vi "UHR-Fleezers Control (fpga) - Leonardo 04-2018 V5.3.vi"() -> ()   [LabVIEW 2013]
doc: "UHR-Fleezers Instrument Control Code (fpga)"
uses:
  <vilib>/Platform/TimedLoop/XDataNode/timing_clust.ctl
  <vilib>/Platform/TimedLoop/XDataNode/nitl_modes.ctl
  <vilib>/Platform/TimedLoop/XDataNode/wakeup.ctl
  <vilib>/rvi/eio/common/nirviEmuTemplateMethod_errors.vi
  <vilib>/rvi/Emulation/niFpgaSctlEmulationGetInTimedLoop.vi
  <vilib>/rvi/Emulation/niFpgaEmulationReportErrorSimple.vi
  <vilib>/rvi/Emulation/niFpgaGetClockAttributes.vi
  <vilib>/rvi/Emulation/niFpgaCriticalErrorInLSC.vi
  <vilib>/rvi/FIFO/Fifo_Resource/nirvififoEmulationReadFpgaImpl.vi
  <vilib>/rvi/DataTransferAndStorage/Container/Common/niFpgaContainerGetUniqueNameForEmu.vi
  <vilib>/rvi/DataTransferAndStorage/Container/Common/niFpgaContainerExecOnDevCompGetState.vi
  <vilib>/rvi/interface/RandomDataEmulation/nirviRandomDataFPGAFIFO.vi
  <vilib>/rvi/interface/RandomDataEmulation/niFpgaRandomDataHandleErrors.vi
  <vilib>/rvi/eio/common/nirviEmuReportErrorAndStop.vi
  <vilib>/rvi/Emulation/niFpgaProcessEmulError.vi
  <vilib>/rvi/FIFO/Fifo_Resource/nirvififoEmulationWriteFpgaImpl.vi
  <vilib>/Platform/TimedLoop/XDataNode/XDataNode.xnode
  <vilib>/eio/EIOMethodNode/EIOMethodNode.xnode
  <vilib>/eio/EIONode/EIONode.xnode
  <vilib>/rvi/DataTransferAndStorage/Container/XNode/niFpgaContainer.xnode
  <vilib>/rvi/FIFO/Fifo_Resource/nirvififoEmulationRead.vi
  <vilib>/rvi/FIFO/Fifo_Resource/niFpgaFifoEmulationRefIn.vi
  <vilib>/rvi/interface/RandomDataEmulation/nirviRandomDataFpgaReadWriteTemplate.vi
  <vilib>/rvi/FIFO/Fifo_Resource/nirvififoEmulationWrite.vi
  <vilib>/addons/control/pid/fpga.llb/XNode/niFpgaPID.xnode
  <vilib>/Platform/TimedLoop/XDataNode/XDNodeRunTimeDep.lvlib
  <vilib>/rvi/Memory/Memory_Emulation/niFpgaMemoryEmulationRefIn.vi
panel:
  in  "Tab Control 2":T1(tab)
  out "BD1 amplitude 1 out":u16
  out "BD1 amplitude 2 out":u16
  in  "FB output range":cluster{"output low":i16, "output high":i16}={"output low"=0, "output high"=3000}
  in  "FB Gains":T2={"proportional gain (Kc)"=10, "integral gain (Kc*Ts/Ti)"=5, "derivative gain (Kc*Td/Ts)"=0}
  in  "RF synth green feedback max":i16=4000
  in  "RD":bool=TRUE
  in  "Swap F1 and F2":bool
  in  "Scan BD":bool
  in  "Start scan":bool
  in  "OSK Bd 1":bool
  in  "Reset Bd 1":bool
  in  "PMODE":bool=TRUE
  in  "Number Interlace Cycles":u8=2 min=1 max=3
  in  "Interlace Off Parameters":u8=1 min=1 max=3
  in  "Interlace ON/OFF":bool
  out "DIO Relative phase":i16
  in  "Phase count adjustment (DIO)":i16
  in  "+ phase (DIO)":bool
  out "DIO Late Counter":u8
  in  "DIO count 1 (ticks)":u16=400
  in  "DIO count 2 (ticks)":u16=400
  in  "DIO count 3 (ticks)":u16=400
  out "AI2 Y Sum Set 2":i16
  out "AI2 Y Sum Set 1":i16
  in  "FB Setpoint Set 1":i16 min=0 step=1
  in  "FB Reset Set 1":bool
  in  "FB On/Off Set 1":bool
  in  "FB Reset Set 2":bool
  in  "FB On/Off Set 2":bool
  in  "FB Setpoint Set 2":i16 min=0 step=1
  in  "Amp switch delay":u8=5
  in  "RF synth bd controls green":bool
  in  "Phase Trap 2":fxp<+,14,14>
  in  "Phase Trap 1":fxp<+,14,14>
  in  "Phase offset method":u8
  in  "BD 2 Amplitude 1":u16
  in  "BD 1 Amplitude 1":u16
  in  "BD 2 Frequency 1":u64
  in  "BD 1 Frequency 1":u64
  in  "BD 2 Amplitude 2":u16
  in  "BD 1 Amplitude 2":u16
  in  "BD 2 Frequency 2":u64
  in  "BD 1 Frequency 2":u64
  in  "BD 2 Amplitude 3":u16
  in  "BD 1 Amplitude 3":u16
  in  "BD 2 Frequency 3":u64
  in  "BD 1 Frequency 3":u64
  in  "BD 2 Delay (Ticks)":u8 caption="Count(Ticks)"
  in  "Next trap write delay (ticks)":u8 caption="Count(Ticks)"
  out "Random phase generated":fxp<+,14,14>
  in  "RF phase reset before cycles":bool
  in  "Trap 1 osc enable":bool
  in  "N trap osc periods":i16
  in  "Trap osc period (pts)":i16
  in  "Osc traps":bool
  in  "Initiate trap osc":bool
  in  "Ready Write":bool
  in  "Data":i64
  in  "Address 2":u32
  in  "Osc trap cont.":bool
  in  "Trap 2 osc enable":bool
  out "green FB running":bool
  in  "APD 2 AO scale factor":i16=1
  in  "BD 1 Delay (ticks)":u8
  in  "Tab Control":T3(tab)=enum."MCL trap control"
  in  "Set 3":bool
  in  "Set 2":bool=TRUE
  in  "Set 1":bool=TRUE
  in  "Trap Pos to FIFO":bool
  in  "N of AI1 Int Acq Sets":i16=2 min=1 max=3 step=1
  out "AI Late Counter":u8
  in  "ai count":u16=400
  in  "+ phase":bool
  in  "Phase count adjustment":i16
  out "Relative phase":i16
  in  "AI to FIFO":bool
  out "BD1 Frequency Out 1":u64
  out "BD1 Frequency Out 2":u64
  out "Trap Pos FIFO Timeout":u16
  out "Trap AI FIFO Timeout":u16
  in  "Trap FIFO Set Timeout":i32
  in  "Scan freq.  increment":i64
  in  "Scan steps":u64
  in  "Number of scans":u16
  in  "Cycles per step":u64
  in  "Raster setpoint":fxp<+/-,16,1>
  in  "Raster to target force":bool
  out "Actual Scan freq":u64
  in  "Cont. Scan":bool
  out "Scan I":u64
  in  "Abort scan":bool
  out "Scanning":bool
  in  "Symmetric FB/Raster":bool
  in  "FB Min frequency":u64
  in  "FB Max Frequency":u64
  in  "Dynamic Force FB (Ronen)":bool
  in  "Trap pos. FB Range":T4={"FB2 output low"=-1.0, "FB2 output high"=0.999969482421875}
  in  "Trap Pos. FB Gains":T5={"proportional gain (Kc)"=0.999969482421875, "integral gain (Kc*Ts/Ti)"=0.999969482421875, "derivative gain (Kc*Td/Ts)"=0.0}
  in  "B factor":fxp<+/-,32,16>
  in  "Negate Diff?":bool
  in  "Diff FB Measurement?":bool
  in  "FB Trig Integrate":u32=1
  out "TTrig?":bool
  in  "TTrig Negate Pos":bool=TRUE
  out "Trap Pos FB Int Signal":fxp<+/-,24,9> format="%.18g"
  out "Trap Pos FB Int-Norm Signal":fxp<+/-,16,1> format="%.16g"
  in  "FPGA TTrig Thresh":i64
  in  "FPGA Trap Trig":bool
  out "Trap Pos FB Action":i64
  in  "Trap Pos. FB Offset Factor":i64
  in  "Trap Pos. FB Mult Factor":i64=2
  in  "Trap Pos. FB Reset":bool
  in  "Trap Pos FB Monitor T1 or T2":bool
  in  "AI1 X Scale":u16
  in  "Trap Pos FB Int Count":u16=100
  in  "Trap Pos FB Negate Action":bool
  out "AI1 X Set 2":fxp<+/-,16,1>
  out "AI1 X Set 1":fxp<+/-,16,1>
  in  "Trap Pos. FB SP":fxp<+/-,16,1>
  in  "Force feedback":bool
  out "TTrig Sig":i64
  out "TTrig Fin Thresh":i64
  in  "1D or 2D Scan?":bool
  in  "Abort scan (MCL)":bool
  in  "MCL Scan Axis":bool
  in  "Cont. Scan (MCL)":bool
  out "Scan I (MCL)":u64
  in  "Number of scans (MCL)":u16
  out "Scanning MCL":bool
  in  "Scan steps (MCL)":u64
  in  "Cycles per step (MCL)":u64
  in  "Scan freq.  increment (MCL)":i16
  in  "Start scan (MCL)":bool
  in  "AO2 (X)":i16
  in  "AO1 (Y)":i16
  out "MCL Late Counter":u8
  in  "MCL count":u32=800
  out "MCL Relative Phase":i16
  in  "Phase count adjustment (MCL)":i16
  in  "+ phase (MCL)":bool
  in  "Lifetime events to read blue":u16=100
  in  "Lifetime read blue fifo":bool
  out "lifetime events in fifo":u16
  out "APD2 int gate":bool
  in  "APD Gate Operating Mode":u8 max=2 step=1
  in  "Invert APD Gate":bool
  in  "APD Gate OFF Count":u16=100
  in  "APD Gate ON Count":u16=300
  out "APD 1 Gate Late Counter":u8
  out "APD 1 Gate Relative Phase":i16
  in  "Phase count adjustment (APD 1 Gate)":i16
  in  "+ phase (APD 1 Gate)":bool
  out "APD 2 Counts 0":u32
  out "APD 2 Counts 1":u32
  out "APD 1 Counts 0":u32
  out "APD 1 Counts 1":u32
  in  "Phase count adjustment (APD 2 Gate)":i16
  out "APD 2 Gate Late Counter":u8
  out "APD 2 Gate Relative Phase":i16
  in  "+ phase (APD 2 Gate)":bool
  out "APD 3 Counts 0":u32
  out "APD 3 Counts 1":u32
  out "APD 3 Gate Late Counter":u8
  in  "Phase count adjustment (APD 3 Gate)":i16
  out "APD 3 Gate Relative Phase":i16
  in  "+ phase (APD 3 Gate)":bool
  out "APD1 int gate":bool
  out "APD3 int gate":bool
  in  "Lifetime timeout APD1":u16=200
  in  "APD to FIFO":bool
  in  "APD Acq Rate Count":u32=20000000
  out "APD Acq Late Counter":u16
  out "APD Acq Relative Phase":i16
  in  "+ phase (APD Acq)":bool
  in  "Phase Count Adjustment (APD Acq)":i16
  in  "APD 1 AO scale factor":i16=1
  out "APD2 out state":bool
  out "APD1 out state":bool
  out "APD Acq Late?":bool
  in  "Number of OFF cycles":i16
  in  "Green long-scale interlacing":bool
  in  "D3 2":i16
  in  "I3 2":i16=5
  in  "P3 2":i16=10
  in  "Green FB Setpoint 2":i16=250 min=0 step=1
  in  "Green FB Reset 2":bool
  in  "Green Filter Flipper":bool
  in  "Green interlace OFF count":u16=100
  out "GI Relative phase":i16
  in  "Phase count adjustment (GI)":i16
  in  "+ phase (GI)":bool
  in  "Green interlace ON count":u16=300
  out "GI Late Counter":u8
  in  "Invert GI":bool
  in  "Operating Mode":u8 max=2 step=1
  in  "Current Out":u16=30000
  in  "Green int current ON count adj":u32=150
  in  "Green interlace OFF count 2":u32=900
  in  "Green interlace ON count 2":u32=300
  out "GI Late Counter 2":u16
  in  "Green FB Count":u32=1200
  in  "Phase count adjustment (GI) 2":i16=20
  in  "Green FB Setpoint":i16=250 min=0 step=1
  in  "Invert GI 2":bool
  out "GI Relative phase 2":i16
  in  "+ phase (GI) 2":bool
  in  "Phase count adjustment (Green FB)":i16=10
  out "Green Late Counter":u16
  out "Green FB Relative Phase":i16
  in  "+ phase (Green FB)":bool
  out "Green FB Signals":T6
  out "Green FB Sum":i16
  in  "Green FB Gains":T2={"proportional gain (Kc)"=10, "integral gain (Kc*Ts/Ti)"=5, "derivative gain (Kc*Td/Ts)"=0}
  in  "Green FB On/Off":bool
  in  "Green FB Reset":bool
  out "Green FB Late?":bool
  out "GI Late?":bool
  in  "Operating Mode 2":u8=2 max=2 step=1
  in  "Chassis2/Mod4/AO1":u16
  in  "Number of ON cycles":i16
  in  "+ phase (RI)":bool
  out "RI Relative phase":i16
  out "RI Late Counter":u8
  in  "Red interlace ON count":u16=300
  in  "Red interlace OFF count":u16=100
  in  "Invert RI":bool
  in  "Red Laser Operating Mode":u8 max=2 step=1
  in  "Phase count adjustment (RI)":i16
  in  "Phase count adjustment (BI D)":i16
  in  "Blue Laser Operating Mode (D)":u8 max=2 step=1
  in  "Invert BI (D)":bool
  in  "Blue interlace OFF count (D)":u16=100
  in  "Blue interlace ON count (D)":u16=300
  out "Blue Late Counter (D)":u8
  out "BI Relative phase (D)":i16
  in  "+ phase (BI D)":bool
  in  "Lifetime to FIFO":bool
  out "lifetime (ticks)":u16
  # "Raster Scan AOD"
  # "1 (X)"
  # "2 (Y)"
  # "IR Intensity Feedback (RF BD 1)"
  # "FB Gains Set 1"
  # "FB output range 1"
  # "IR Intensity Feedback (RF BD 2) -\nonly when using BD 2 for green laser AOM (not trap Y)"
  # "Keep below 4096 (12 bits) to stay within range of RF board. Going over doesn't saturate, it truncates higher bits."
  # "RF phase offset control"
  # "Methods are:\n0 - Default, do nothing at all (no phase offset writes)\n1 - Manual phase adjustment\n2 - Cycle the phase adjustment using the input phase numbers as increment values for each cycle"
  # "False is usual, True is external loop method"
  # "Parameters if using the external RF switching loop"
  # "Parameters if using the usual internal RF switching method"
  # "FB Triggering Excitation Laser"
  # "Trap Pos. FB Gains"
  # "Trap Pos. FB Range"
  # "AO1 (Y)"
  # "2D"
  # "Trap 3"
  # "1D"
  # "AO2 (X)"
  # "Fl Laser"
  # "APD AO for aligning"
  # "Detection Loop"
  # "Green fluorescent laser digital gate interlacing loop"
  # "0 Forced ON\n1 Forced OFF\n2 Interlacing"
  # "ALEX settings:"
  # "Controls for usual IA ME controls green AOM"
  # "Controls for RF synth board controls green AOM"
  # "Green FB Gains"
  # "Red fluorescent laser digital gate interlacing loop"
  # "Detection Loop"
  # "0 Forced ON\n1 Forced OFF\n2 Interlacing"
  # "Analog/FB Control Loop\n(Disabled)"
  # "Digital Control Loop"
  # "Blue laser intensity reading"
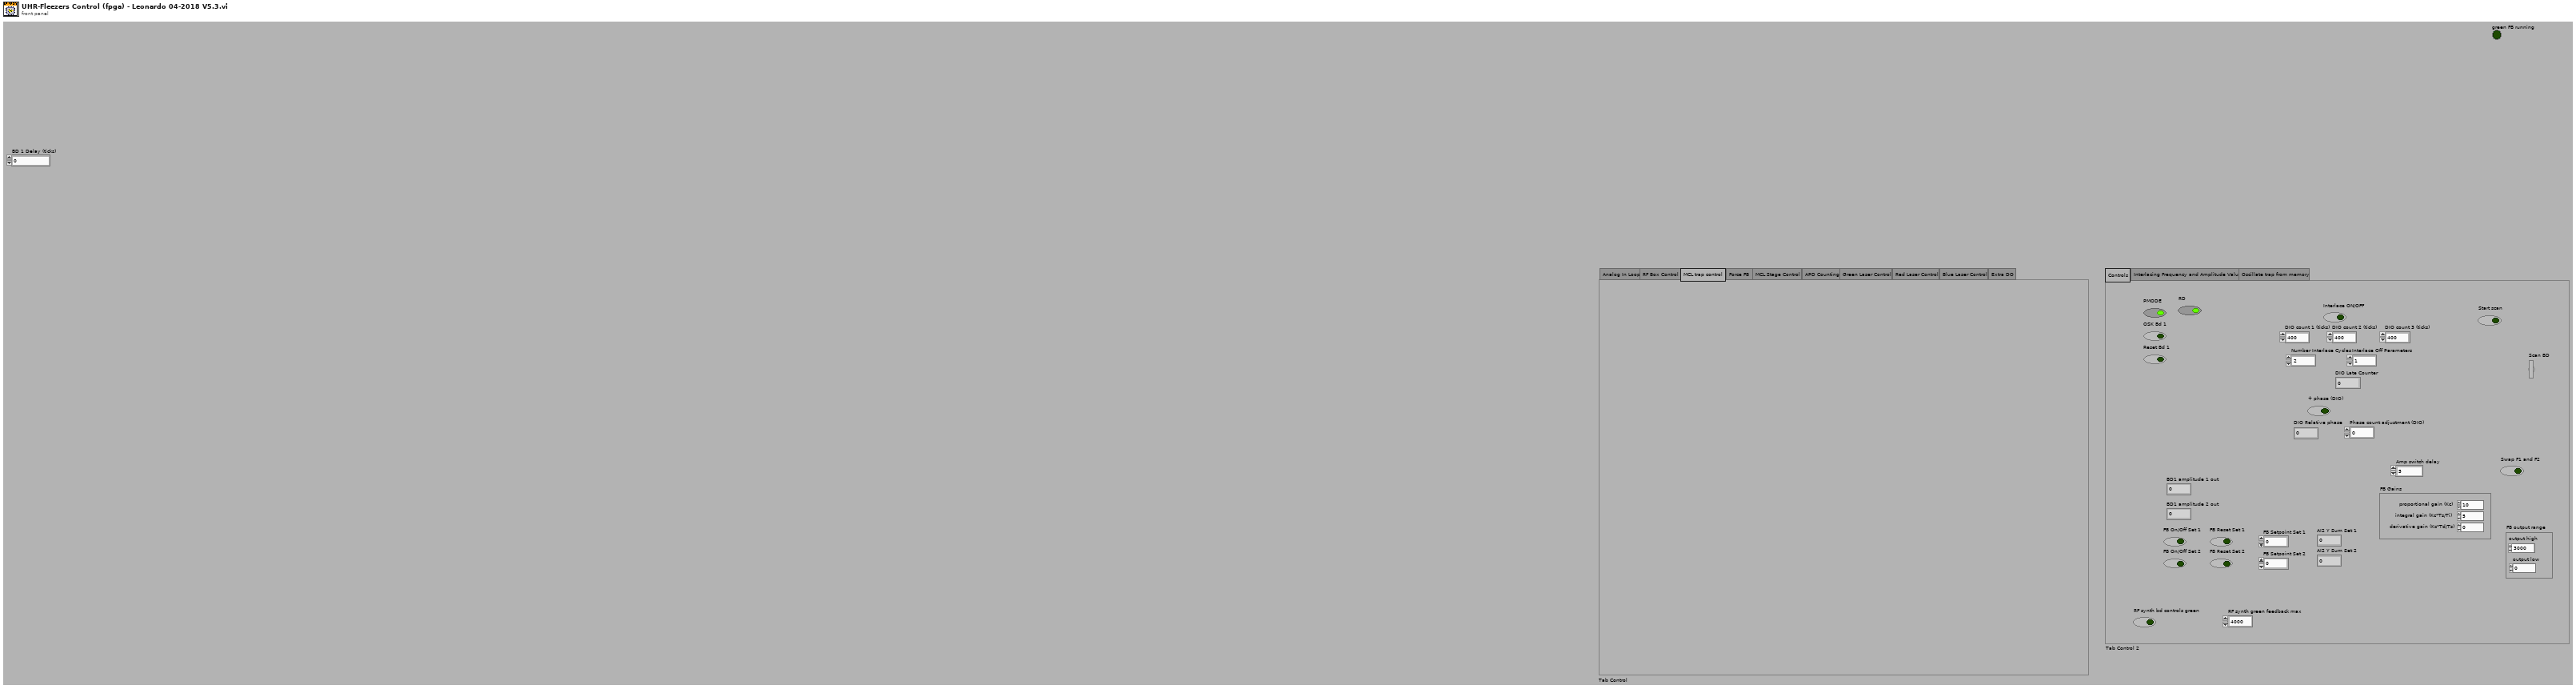
[diagram p1: front panel]
types:
  T1 = enum32{"Controls", "Interlacing Frequency and Amplitude Values", "Oscillate trap from memory"}
  T2 = cluster{"proportional gain (Kc)":i16, "integral gain (Kc*Ts/Ti)":i16, "derivative gain (Kc*Td/Ts)":i16}
  T3 = enum32{"Analog In Loop", "RF Box Control", "MCL trap control", "Force FB", "MCL Stage Control", "APD Counting", "Green Laser Control", "Red Laser Control", "Blue Laser Control", "Extra DO"}
  T4 = cluster{"FB2 output low":fxp<+/-,16,1>, "FB2 output high":fxp<+/-,16,1>}
  T5 = cluster{"proportional gain (Kc)":fxp<+/-,16,1>, "integral gain (Kc*Ts/Ti)":fxp<+/-,16,1>, "derivative gain (Kc*Td/Ts)":fxp<+/-,16,1>}
  T6 = cluster{"Green FB Ch 0":i16, "Green FB Ch 1":i16, "Green FB Ch 2":i16}
  T7 = typedef "XDNodeRunTimeDep.lvlib/timing_clust.ctl" = cluster{"Expected End [f-1]":u64, "Actual End [f-1]":u64, "Finished Late? [f-1]":bool, "Expected End [i-1]":u64, "Actual End [i-1]":u64, "Finished Late? [i-1]":bool, "Expected Start [i]":u64, "Actual Start [i]":u64, "Expected Start [f]":u64, "Actual Start [f]":u64, "Source Name":string, "Structure Name":string, "Period":i64, "Deadline":i64, "Offset":i64, "Start":i64, "Priority":i32, "Timeout":i32, "Mode":T8, "Wakeup Reason":T9, "Error":errorcluster, "Source Type":string, "Secondary Source Type":string, "Global End Time":u64, "Global Start Time":u64, "Frame Duration":u64, "Iteration Duration":u64, "Assigned CPU":i32, "I/O Scan Engine Mode":u32}
  T8 = typedef "XDNodeRunTimeDep.lvlib/nitl_modes.ctl" = enum32{"No Change", "Process missed periods, maintain original phase", "Discard missed periods, maintain original phase", "Process missed periods, ignore original phase", "Discard missed periods, ignore original phase"}
  T9 = typedef "XDNodeRunTimeDep.lvlib/wakeup.ctl" = enum32{"Normal", "Aborted", "Asynchronous wakeup", "Timing source error", "Timed loop error", "Timeout"}
  T10 = cluster{"Chassis2/Mod2/AI0":i16, "Chassis2/Mod2/AI1":i16, "Chassis2/Mod2/AI2":i16}
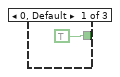
[diagram p2: hidden frame]
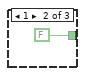
[diagram p3: hidden frame]
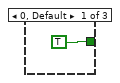
[diagram p6: hidden frame]
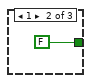
[diagram p7: hidden frame]
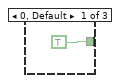
[diagram p11: hidden frame]
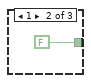
[diagram p12: hidden frame]
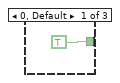
[diagram p13: hidden frame]
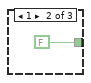
[diagram p14: hidden frame]
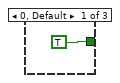
[diagram p18: hidden frame]
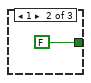
[diagram p19: hidden frame]
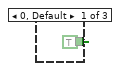
[diagram p20: hidden frame]
diagram:
  w5 = FALSE
  w6 = FALSE
  # "BD2 amp"
  # "BD1 amp"
  # "BD2 amp"
  # "BD1 amp"
  # "timing array current index"
  # "timing array"
  # "timing counter (phase adjusted here)"
  # "late counter"
  n1 = while {
    stop <- FALSE stop-if-true
    n2 = xnode "FPGA I/O Node"("Connector0/DIO3"="Green Filter Flipper", "Chassis2/Mod1/AO1"="Chassis2/Mod4/AO1") -> ()  [unwired: 2 in, 2 out]
    n3 = call "Loop Timer11"("Count(Ticks)"=u32 40000 ("Extra DO Counts")) -> ()  [unwired: 1 out]
  }
  n4 = disable-structure shown="Disabled" {
    frame Disabled {
      w20 = i16 2 items=["UnSet Ready", "ReadWrite", "Wait Ready"]
      n5 = while "Handshake memory transfer for trap oscillation sin wave data" {
        shift-right: [w22] -> _
        shift-left: w20 -> [w23]
        stop <- FALSE stop-if-true
        # "Write"
        n6 = case shown="1" w23 {
          tunnel: [w26 w31 w32] -> w22
          frame 3, Default {
            w24 = i16 2 items=["UnSet Ready", "ReadWrite", "Wait Ready"]
            w25 = i16 1 items=["UnSet Ready", "ReadWrite", "Wait Ready"]
            n7 = Select(t=w25, s="Ready Write", f=w24) -> (s? t:f=w26:i16)
          }
          frame 1 {
            w31 = i16 0 items=["UnSet Ready", "ReadWrite", "Wait Ready"]
            n8 = xnode ("Memory Write")("Address"="Address 2", "Data"="Data", "Memory In"=refnum<k21> "Trap osc memory") -> ()  [unwired: 1 out]
          }
          frame 0 {
            w32 = i16 2 items=["UnSet Ready", "ReadWrite", "Wait Ready"]
            n9 = local write "Ready Write"(FALSE ("Ready Read")) -> ()
          }
        }
      }
    }
    frame Enabled {
    }
  }
  n10 = flat-sequence "FPGA initialization to do before running any of the loops" {
    tunnel: [u16 0 ("DIO count 3 (ticks)")] -> w4
    tunnel: [w41] -> _
    frame #0 {
      # "UDCLK out enable and set low"
      # "WR"
      # "BD 2"
      # "BD 1"
      # "With the RF synth board initialization now done in a separate fpga vi, now when this vi is started, board is already configured and is ready for interlacing. Just need to set WR high and enabled UDCLK as write and set to low.\nbefore setting data and address bits."
      # "Start up expansion chassis early\nto avoid delays later"
      # "Set data and address values to something safe (a correct setting) so any initial WR and udclk flipping doesn't have a chance to mess anything up. Safe would be setting an unused data entry:"
      n11 = xnode "FPGA I/O Method Node"("Enable"=TRUE) -> ("FPGA I/O Out"=w35:refnum<k21>)  [unwired: 1 in]
      n12 = xnode "FPGA I/O Method Node"("Enable"=TRUE) -> ("FPGA I/O Out"=w38:refnum<k21>)  [unwired: 1 in]
      n13 = xnode "FPGA I/O Node"("Chassis2/Mod1/AO0"=u16 0 ("Chassis2/Mod4/AO0")) -> ("Chassis2/Mod2/AI0"=w41:i16)  [unwired: 2 in, 2 out]
      n14 = xnode "FPGA I/O Node"("Connector1/DIO15"=TRUE) -> ()  [unwired: 1 in, 1 out]
      n15 = xnode "FPGA I/O Node"("I/O Item"=FALSE ("Connector1/DIO30"), "FPGA I/O In"=w35) -> ()  [unwired: 1 out]
      n16 = xnode "FPGA I/O Node"("I/O Item"=FALSE ("Connector1/DIO30"), "FPGA I/O In"=w38) -> ()  [unwired: 1 out]
      n17 = xnode "FPGA I/O Node"("Connector1/DIO0"=FALSE, "Connector1/DIO1"=FALSE, "Connector1/DIO2"=FALSE, "Connector1/DIO3"=FALSE, "Connector1/DIO4"=FALSE, "Connector1/DIO5"=FALSE, "Connector1/DIO6"=FALSE, "Connector1/DIO7"=FALSE, "Connector1/DIO8"=FALSE, "Connector1/DIO9"=FALSE, "Connector1/DIO10"=FALSE, "Connector1/DIO11"=FALSE, "Connector1/DIO12"=FALSE, "Connector1/DIO13"=FALSE, "Connector1/DIO20"=FALSE, "Connector1/DIO21"=FALSE, "Connector1/DIO22"=FALSE, "Connector1/DIO23"=FALSE, "Connector1/DIO24"=FALSE, "Connector1/DIO25"=FALSE, "Connector1/DIO26"=FALSE, "Connector1/DIO27"=FALSE, "Connector1/DIO14"=FALSE) -> ()  [unwired: 23 in, 23 out]
    }
  }
  n18 = node-c288() -> (w12:T7)  [unwired: 1 in]
  n19 = timed-loop "RF box board DIO control: control bits" {
    timing: w12 -> [_]
    timing-out: [_] -> w11
    tunnel: [w68] -> _
    tunnel: w4 -> [w68]
    stop <- FALSE stop-if-true
    n20 = xnode "FPGA I/O Node"("Connector1/DIO16"="RD", "Connector1/DIO17"="PMODE", "Connector1/DIO18"="OSK Bd 1", "Connector1/DIO19"="Reset Bd 1") -> ()  [unwired: 4 in, 4 out]
  }
  n21 = node-c288(w11) -> ()
  n22 = local read "AO1 (Y)"() -> (w14:i16)
  n23 = local read "AO2 (X)"() -> (w13:i16)
  n24 = To Unsigned Long Integer(number=w4) -> (unsigned 32bit integer=w7:u32)
  n25 = disable-structure shown="Disabled" {
    disable-tunnel: w6 -> [w76 _]
    disable-tunnel: w4 -> [w75 _]
    frame Disabled {
      n26 = while "APD 2 Gating" {
        shift-right: [w80] -> _
        shift-left: w75 -> [w85]
        shift-right: [w79] -> _
        shift-left: w76 -> [w77]
        stop <- FALSE stop-if-true
        n27 = flat-sequence {
          tunnel: w85 -> [w88]
          tunnel: [w89] -> w83
          tunnel: [w88] -> w81
          tunnel: [w87] -> w78
          tunnel: w77 -> [w87]
          tunnel: [w92] -> w84
          tunnel: w83 -> [w92]
          tunnel: [w91] -> w82
          tunnel: w81 -> [w91]
          tunnel: w78 -> [w90]
          tunnel: [w114] -> w80
          tunnel: w84 -> [w124]
          tunnel: w82 -> [w122]
          tunnel: [w93] -> w79
          frame #0 {
            n28 = call "Loop Timer3"("Count(Ticks)"=w88) -> ("Tick Count(Ticks)"=w89:u32)
          }
          frame #1 {
            # "Signal maybe then sent through \na transistor before APD"
            n29 = xnode "FPGA I/O Node"("Connector1/DIO34"=w90) -> ()  [unwired: 1 in, 1 out]
            "APD2 int gate" <- w90
          }
          frame #2 {
            n30 = local read "APD Gate ON Count"() -> (w107:u16)
            n31 = local read "APD Gate OFF Count"() -> (w106:u16)
            n32 = feedback #1(TRUE) -> (w119:bool)
            n33 = feedback-in #2(w124) -> ()
            n34 = feedback #2(w124) -> (w108:u32)
            n35 = Not(x=w119) -> (.not. x?=w117:bool)
            n36 = feedback-in #1(w117) -> ()
            n37 = Subtract(x=w124, y=w108) -> (x-y=w123:u32)
            n38 = Select(t=w107, s=w117, f=w106) -> (s? t:f=w121:u16)
            n39 = Subtract(x=w123, y=w122) -> (x-y=w99:u32)
            n40 = Subtract(x=w121, y=w99) -> (x-y=w113:u32)
            n41 = Number To Boolean Array(number=w99) -> (Boolean array=w98:bool[])
            n42 = Or Array Elements(Boolean array=w98) -> (logical OR=w97:bool)
            n43 = Boolean To (0,1)(Boolean="+ phase (APD 2 Gate)") -> (0, 1=w111:i16)
            n44 = Multiply(x=w111, y="Phase count adjustment (APD 2 Gate)") -> (x*y=w109:i16)
            n45 = Boolean To (0,1)(Boolean=w97) -> (0, 1=w104:i16)
            n46 = Add(x=w113, y=w109) -> (x+y=w114:u32)
            n47 = To Unsigned Byte Integer(number=w104) -> (unsigned 8bit integer=w101:u8)
            n48 = feedback #3(i16 0) -> (w116:i16)
            n49 = Subtract(x=w116, y=w109) -> (x-y=w115:i16)
            "APD 2 Gate Relative Phase" <- w115
            n50 = feedback-in #3(w115) -> ()
            n51 = feedback #4(u8 0) -> (w102:u8)
            n52 = Add(x=w101, y=w102) -> (x+y=w100:u8)
            "APD 2 Gate Late Counter" <- w100
            n53 = feedback-in #4(w100) -> ()
            n54 = local read "APD Gate Operating Mode"() -> (w105:u8)
            n55 = case shown="2" w105 {
              tunnel: [TRUE FALSE w127] -> w94
              tunnel: w119 -> [_ _ w127]
              frame 0, Default {
              }
              frame 1 {
              }
              frame 2 {
              }
            }
            n56 = local read "Invert APD Gate"() -> (w96:bool)
            n57 = Not(x=w94) -> (.not. x?=w95:bool)
            n58 = Select(t=w95, s=w96, f=w94) -> (s? t:f=w93:bool)
          }
        }
      }
    }
    frame Enabled {
    }
  }
  n59 = while "DAQ AI set 1" {
    shift-right: [w128] -> _
    shift-left: w4 -> [w133]
    stop <- FALSE stop-if-true
    n60 = flat-sequence {
      tunnel: w133 -> [w144]
      tunnel: [w143] -> w131
      tunnel: [w144] -> w130
      tunnel: [w154] -> w141
      tunnel: [w153] -> w140
      tunnel: [w152] -> w139
      tunnel: [w151] -> w138
      tunnel: [w150] -> w137
      tunnel: [w149] -> w136
      tunnel: [w148] -> w135
      tunnel: [w147] -> w134
      tunnel: [w146] -> w132
      tunnel: w131 -> [w146]
      tunnel: w130 -> [w145]
      tunnel: [w145] -> w129
      tunnel: [w184] -> w128
      tunnel: w141 -> [w210]
      tunnel: w140 -> [w176]
      tunnel: w139 -> [w177]
      tunnel: w138 -> [w156]
      tunnel: w137 -> [w200]
      tunnel: w136 -> [w199]
      tunnel: w135 -> [w198]
      tunnel: w134 -> [w197]
      tunnel: w132 -> [w194]
      tunnel: w129 -> [w191]
      frame #0 {
        n61 = call "Loop Timer"("Count(Ticks)"=w144) -> ("Tick Count(Ticks)"=w143:u32)
      }
      frame #1 {
        n62 = xnode "FPGA I/O Node"("Connector1/DIO31"=TRUE ("Connector1/DIO33")) -> ("Connector0/AI0"=w154:i16, "Connector0/AI1"=w153:i16, "Connector0/AI2"=w152:i16, "Connector0/AI3"=w151:i16, "Connector0/AI4"=w150:i16, "Connector0/AI5"=w149:i16, "Connector0/AI6"=w148:i16, "Connector0/AI7"=w147:i16)  [unwired: 9 in, 9 out]
      }
      frame #2 {
        w180 = FALSE ("AI to FIFO")
        # "Normalize by trap bead QPD sum, AI3"
        # "Adjust phase after data acquired if button pressed"
        n63 = feedback #5(i16 1) -> (w203:i16)
        n64 = Increment(x=w203) -> (x+1=w209:i16)
        n65 = Scale By Power Of 2(n="AI1 X Scale", x=w176) -> (x*2^n=w174:i16)
        n66 = Greater?(x=w209, y="N of AI1 Int Acq Sets") -> (0:w206:bool)
        n67 = Select(t=i16 1, s=w206, f=w209) -> (s? t:f=w208:i16)
        n68 = feedback-in #5(w208) -> ()
        n69 = Divide(x=w174, y=w156) -> (x/y=w173:fxp<+/-,16,1>)
        n70 = feedback #6(w180) -> (w178:bool)
        n71 = feedback #7(w180) -> (w196:bool)
        n72 = case shown="1, Default" w203 {
          tunnel: w177 -> [w233 w240 _]
          tunnel: ["Set 1" "Set 2" "Set 3"] -> w201
          tunnel: ["AI to FIFO" w242 w247] -> w195
          tunnel: w196 -> [_ w242 w247]
          tunnel: ["Trap Pos to FIFO" w241 w246] -> w179
          tunnel: w178 -> [_ w241 w246]
          tunnel: w173 -> [w232 w239 _]
          tunnel: [w231 w237 FALSE] -> w160
          tunnel: [w230 w238 u64 0 ("BD1 Frequency Out 2")] -> w159
          frame 1, Default {
            n73 = local read "BD1 Frequency Out 1"() -> (w230:u64)
            n74 = Compound Arithmetic op=AND("Trap Pos to FIFO", "Set 1", "AI to FIFO") -> (w231:bool)
            "AI2 Y Sum Set 1" <- w233
            "AI1 X Set 1" <- w232
          }
          frame 2 {
            n75 = local read "BD1 Frequency Out 2"() -> (w238:u64)
            n76 = Compound Arithmetic op=AND(w241, "Set 2", w242) -> (w237:bool)
            "AI2 Y Sum Set 2" <- w240
            "AI1 X Set 2" <- w239
          }
          frame 3 {
          }
        }
        n77 = And(x=w201, y=w195) -> (x .and. y?=w202:bool)
        n78 = case shown="True" w202 {
          tunnel: w210 -> [_ w261]
          tunnel: w176 -> [_ w260]
          tunnel: w177 -> [_ w259]
          tunnel: w156 -> [_ w258]
          tunnel: w200 -> [_ w257]
          tunnel: w199 -> [_ w256]
          tunnel: w198 -> [_ w255]
          tunnel: w197 -> [_ w254]
          tunnel: 0 ("DMA buffer timeout") -> [_ w263]
          frame False {
          }
          frame True {
            n79 = Build Array(w261, w260, w259, w258, w257, w256, w255, w254) -> (w262:i16[])
            n80 = for {
              tunnel: w262 -> [w265] mode=indexing
              tunnel: w263 -> [w266]
              tunnel: [w264] -> w252 mode=indexing
              n81 = xnode ("FIFO Write")("Element"=w265, "Timeout"=w266) -> ("Timed Out?"=w264:bool)  [unwired: 1 in, 1 out]
            }
            n82 = Or Array Elements(Boolean array=w252) -> (logical OR=w249:bool)
            n83 = Boolean To (0,1)(Boolean=w249) -> (0, 1=w251:i16)
            n84 = feedback #8(u16 0) -> (w250:u16)
            n85 = Add(x=w251, y=w250) -> (x+y=w248:u16)
            "Trap AI FIFO Timeout" <- w248
            n86 = feedback-in #8(w248) -> ()
          }
        }
        n87 = feedback-in #6(w179) -> ()
        n88 = feedback-in #7(w195) -> ()
        n89 = case shown="True" w160 {
          tunnel: w159 -> [_ w216]
          tunnel: [u8 0 w213] -> w158
          frame False {
          }
          frame True {
            n90 = Split Number(x=w216) -> (hi(x)=w217:u32, lo(x)=w218:u32)
            n91 = Split Number(x=w217) -> (lo(x)=w219:u16)  [unwired: 1 out]
            n92 = Split Number(x=w218) -> (hi(x)=w220:u16, lo(x)=w221:u16)
            n93 = Build Array "BD 1 nu Stack"(w219, w220, w221) -> (w215:u16[])
            n94 = for {
              tunnel: w215 -> [w228] mode=indexing
              shift-right: [w224] -> w213
              shift-left: u8 0 -> [w225]
              n95 = xnode ("FIFO Method Node")("Element"=w228, "Timeout"="Trap FIFO Set Timeout") -> ("Timed Out?"=w227:bool)  [unwired: 1 in, 1 out]
              n96 = Boolean To (0,1)(Boolean=w227) -> (0, 1=w226:i16)
              n97 = To Unsigned Byte Integer(number=w226) -> (unsigned 8bit integer=w223:u8)
              n98 = Add(x=w223, y=w225) -> (x+y=w224:u8)
            }
          }
        }
        n99 = To Unsigned Word Integer(number=w158) -> (unsigned 16bit integer=w157:u16)
        n100 = feedback #9(u16 0) -> (w171:u16)
        n101 = Add(x=w157, y=w171) -> (x+y=w170:u16)
        "Trap Pos FIFO Timeout" <- w170
        n102 = feedback-in #9(w170) -> ()
        n103 = feedback-in #10(w194) -> ()
        n104 = feedback #10(w194) -> (w193:u32)
        n105 = Subtract(x=w194, y=w193) -> (x-y=w192:u32)
        n106 = xnode "FPGA I/O Node"("Connector1/DIO31"=FALSE ("Connector1/DIO34")) -> ()  [unwired: 1 in, 1 out]
        n107 = Subtract(x=w192, y=w191) -> (x-y=w162:u32)
        n108 = Boolean To (0,1)(Boolean="+ phase") -> (0, 1=w187:i16)
        n109 = Multiply(x=w187, y="Phase count adjustment") -> (x*y=w181:i16)
        n110 = Subtract(x="ai count", y=w162) -> (x-y=w185:u32)
        n111 = Number To Boolean Array(number=w162) -> (Boolean array=w163:bool[])
        n112 = feedback #11(i16 0) -> (w183:i16)
        n113 = Add(x=w185, y=w181) -> (x+y=w184:u32)
        n114 = Subtract(x=w183, y=w181) -> (x-y=w182:i16)
        "Relative phase" <- w182
        n115 = feedback-in #11(w182) -> ()
        n116 = Or Array Elements(Boolean array=w163) -> (logical OR=w161:bool)
        n117 = Boolean To (0,1)(Boolean=w161) -> (0, 1=w168:i16)
        n118 = To Unsigned Byte Integer(number=w168) -> (unsigned 8bit integer=w165:u8)
        n119 = feedback #12(u8 0) -> (w166:u8)
        n120 = Add(x=w165, y=w166) -> (x+y=w164:u8)
        "AI Late Counter" <- w164
        n121 = feedback-in #12(w164) -> ()
      }
    }
  }
  n122 = while "MCL stage control" {
    shift-right: [w279] -> _
    shift-left: w4 -> [w282]
    shift-right: [w272] -> _
    shift-left: w14 -> [w269]
    shift-right: [w271] -> _
    shift-left: w13 -> [w267]
    stop <- FALSE stop-if-true
    n123 = flat-sequence {
      tunnel: w282 -> [w285]
      tunnel: [w284] -> w278
      tunnel: [w285] -> w276
      tunnel: [w287] -> w270
      tunnel: w269 -> [w287]
      tunnel: [w286] -> w268
      tunnel: w267 -> [w286]
      tunnel: w278 -> [w291]
      tunnel: [w291] -> w277
      tunnel: w276 -> [w290]
      tunnel: [w290] -> w275
      tunnel: w270 -> [w289]
      tunnel: w268 -> [w288]
      tunnel: w277 -> [w299]
      tunnel: w275 -> [w298]
      tunnel: [w299] -> w281
      tunnel: [w298] -> w280
      tunnel: [w297] -> w274
      tunnel: [w296] -> w273
      tunnel: [w371] -> w279
      tunnel: w281 -> [w378]
      tunnel: w280 -> [w375]
      tunnel: w274 -> [w373]
      tunnel: w273 -> [w372]
      tunnel: [w373] -> w272
      tunnel: [w372] -> w271
      frame #0 {
        n124 = call "Loop Timer3"("Count(Ticks)"=w285) -> ("Tick Count(Ticks)"=w284:u32)
      }
      frame #1 {
        n125 = xnode "FPGA I/O Node"("Connector0/AO1"=w289, "Connector0/AO2"=w288) -> ()  [unwired: 2 in, 2 out]
      }
      frame #2 {
        n126 = local read "Scanning MCL"() -> (w311:bool)
        n127 = Or(x=w311, y="Start scan (MCL)") -> (x .or. y?=w306:bool)
        n128 = Not(x="Abort scan (MCL)") -> (.not. x?=w304:bool)
        n129 = And(x=w304, y=w306) -> (x .and. y?=w303:bool)
        n130 = case "Raster scan" shown="False" w303 {
          tunnel: [w312 w355] -> w308
          tunnel: "Start scan (MCL)" -> [_ w340]
          tunnel: [w312 w316] -> w292
          frame False {
            w312 = i16 0
            n131 = local write "Scanning MCL"(FALSE ("scanning")) -> ()
          }
          frame True {
            w326 = i16 0
            w325 = u64 0
            # "scan incr."
            # "freq. incr. mult."
            # "count steps"
            # "count number of cycles"
            n132 = feedback #13(w325) -> (w352:u64)
            n133 = Select(t=w325, s=w340, f=w352) -> (s? t:f=w354:u64)
            n134 = Increment(x=w354) -> (x+1=w351:u64)
            n135 = Greater?(x="Cycles per step (MCL)", y=w351) -> (0:w335:bool)
            n136 = Select(t=w351, s=w335, f=w325) -> (s? t:f=w350:u64)
            n137 = feedback-in #13(w350) -> ()
            n138 = feedback #14(w325) -> (w349:u64)
            n139 = Select(t=w325, s=w340, f=w349) -> (s? t:f=w344:u64)
            n140 = Increment(x=w344) -> (x+1=w348:u64)
            n141 = Add(x="Scan steps (MCL)", y="Scan steps (MCL)") -> (x+y=w347:u64)
            n142 = Select(t=w344, s=w335, f=w348) -> (s? t:f=w330:u64)
            n143 = Greater?(x=w347, y=w330) -> (0:w329:bool)
            n144 = Select(t=w330, s=w329, f=w325) -> (s? t:f=w345:u64)
            n145 = feedback-in #14(w345) -> ()
            n146 = Equal?(x="Scan steps (MCL)", y=w330) -> (x = y?=w334:bool)
            n147 = Greater?(x="Scan steps (MCL)", y=w344) -> (0:w343:bool)
            n148 = feedback #15(w326) -> (w346:i16)
            n149 = Select(t=w326, s=w340, f=w346) -> (s? t:f=w332:i16)
            n150 = Increment(x=w332) -> (x+1=w342:i16)
            n151 = Decrement(x=w332) -> (x-1=w341:i16)
            n152 = Select(t=w342, s=w343, f=w341) -> (s? t:f=w333:i16)
            n153 = Select(t=w332, s=w334, f=w333) -> (s? t:f=w331:i16)
            n154 = Select(t=w332, s=w335, f=w331) -> (s? t:f=w327:i16)
            n155 = Select(t=w327, s=w329, f=w326) -> (s? t:f=w328:i16)
            n156 = feedback-in #15(w328) -> ()
            n157 = feedback #16(w325) -> (w339:u64)
            n158 = Select(t=w325, s=w340, f=w339) -> (s? t:f=w314:u64)
            n159 = Increment(x=w314) -> (x+1=w336:u64)
            n160 = Select(t=w314, s=w329, f=w336) -> (s? t:f=w315:u64)
            n161 = Greater?(x="Number of scans (MCL)", y=w315) -> (0:w322:bool)
            n162 = Multiply(x="Scan freq.  increment (MCL)", y=w332) -> (x*y=w355:i16)
            n163 = Select(t=TRUE, s="Cont. Scan (MCL)", f=w322) -> (s? t:f=w321:bool)
            "Scanning MCL" <- w321
            n164 = Select(t=w315, s=w321, f=w325) -> (s? t:f=w337:u64)
            n165 = feedback-in #16(w337) -> ()
            n166 = Increment(x=w315) -> (x+1=→"Scan I (MCL)":u64)
            n167 = To Word Integer(number=w314) -> (16bit integer=w317:i16)
            n168 = Multiply(x=w317, y="Scan freq.  increment (MCL)") -> (x*y=w316:i16)
          }
        }
        n169 = Select(t=w292, s="1D or 2D Scan?", f=i16 0) -> (s? t:f=w293:i16)
        n170 = Select(t=w308, s="MCL Scan Axis", f=w293) -> (s? t:f=w309:i16)
        n171 = Select(t=w293, s="MCL Scan Axis", f=w308) -> (s? t:f=w307:i16)
        n172 = Add(x="AO2 (X)", y=w307) -> (x+y=w296:i16)
        n173 = Add(x="AO1 (Y)", y=w309) -> (x+y=w297:i16)
      }
      frame #3 {
        n174 = feedback-in #17(w378) -> ()
        n175 = feedback #17(w378) -> (w377:u32)
        n176 = Boolean To (0,1)(Boolean="+ phase (MCL)") -> (0, 1=w369:i16)
        n177 = Subtract(x=w378, y=w377) -> (x-y=w376:u32)
        n178 = Multiply(x=w369, y="Phase count adjustment (MCL)") -> (x*y=w365:i16)
        n179 = Subtract(x=w376, y=w375) -> (x-y=w357:u32)
        n180 = Subtract(x="MCL count", y=w357) -> (x-y=w367:u32)
        n181 = feedback #18(i16 0) -> (w366:i16)
        n182 = Subtract(x=w366, y=w365) -> (x-y=w364:i16)
        "MCL Relative Phase" <- w364
        n183 = feedback-in #18(w364) -> ()
        n184 = Number To Boolean Array(number=w357) -> (Boolean array=w358:bool[])
        n185 = Or Array Elements(Boolean array=w358) -> (logical OR=w356:bool)
        n186 = Boolean To (0,1)(Boolean=w356) -> (0, 1=w363:i16)
        n187 = Add(x=w367, y=w365) -> (x+y=w371:u32)
        n188 = To Unsigned Byte Integer(number=w363) -> (unsigned 8bit integer=w360:u8)
        n189 = feedback #19(u8 0) -> (w361:u8)
        n190 = Add(x=w360, y=w361) -> (x+y=w359:u8)
        "MCL Late Counter" <- w359
        n191 = feedback-in #19(w359) -> ()
      }
    }
  }
  n192 = while "APD 2 Counter" {
    tunnel: w4 -> [_]
    stop <- FALSE stop-if-true
    n193 = flat-sequence {
      frame #0 {
        n194 = xnode "FPGA I/O Method Node"("FPGA I/O In"=refnum<k21> "Connector0/DIO1" ("APD 2 DO"), "Timeout"=-1) -> ()  [unwired: 2 out]
      }
      frame #1 {
        n195 = local read "APD1 int gate"() -> (w383:bool)
        n196 = case shown="True" w383 {
          frame False {
          }
          frame True {
            n197 = local read "APD2 out state"() -> (w384:bool)
            n198 = case shown="True" w384 {
              frame False {
                n199 = local read "APD 2 Counts 0"() -> (w386:u32)
                n200 = Increment(x=w386) -> (x+1=→"APD 2 Counts 0":u32)
              }
              frame True {
                n201 = local read "APD 2 Counts 1"() -> (w388:u32)
                n202 = Increment(x=w388) -> (x+1=→"APD 2 Counts 1":u32)
              }
            }
          }
        }
      }
    }
  }
  n203 = while "Green fluorescent laser interlacing (Current to IA 532 nm AOM ME amp)." {
    shift-right: [w394] -> _
    shift-left: w4 -> [w397]
    shift-right: [w391] -> _
    shift-left: i16 0 -> [w389]
    stop <- FALSE stop-if-true
    n204 = flat-sequence {
      tunnel: w397 -> [w400]
      tunnel: [w401] -> w396
      tunnel: [w400] -> w395
      tunnel: [w399] -> w390
      tunnel: w389 -> [w399]
      tunnel: [w404] -> w393
      tunnel: w396 -> [w404]
      tunnel: [w403] -> w392
      tunnel: w395 -> [w403]
      tunnel: w390 -> [w402]
      tunnel: [w417] -> w394
      tunnel: [w433] -> w391
      tunnel: w393 -> [w446]
      tunnel: w392 -> [w443]
      frame #0 {
        n205 = call "Loop Timer10"("Count(Ticks)"=w400) -> ("Tick Count(Ticks)"=w401:u32)
      }
      frame #1 {
        n206 = xnode "FPGA I/O Node"("Chassis2/Mod1/AO0"=w402) -> ()  [unwired: 1 in, 1 out]
      }
      frame #2 {
        n207 = local read "RF synth bd controls green"() -> (w408:bool)
        n208 = Subtract(x="Green interlace OFF count 2", y="Green int current ON count adj") -> (x-y=w426:u32)
        n209 = feedback-in #20(w446) -> ()
        n210 = feedback #20(w446) -> (w445:u32)
        n211 = Add(x="Green int current ON count adj", y="Green interlace ON count 2") -> (x+y=w427:u32)
        n212 = Subtract(x=w446, y=w445) -> (x-y=w444:u32)
        n213 = Subtract(x=w444, y=w443) -> (x-y=w410:u32)
        n214 = Not(x=w408) -> (.not. x?=w406:bool)
        n215 = Number To Boolean Array(number=w410) -> (Boolean array=w411:bool[])
        n216 = Boolean To (0,1)(Boolean="+ phase (GI) 2") -> (0, 1=w423:i16)
        n217 = Or Array Elements(Boolean array=w411) -> (logical OR=w409:bool)
        "GI Late?" <- w409
        n218 = Boolean To (0,1)(Boolean=w409) -> (0, 1=w416:i16)
        n219 = Multiply(x=w423, y="Phase count adjustment (GI) 2") -> (x*y=w419:i16)
        n220 = To Unsigned Word Integer(number=w416) -> (unsigned 16bit integer=w412:u16)
        n221 = feedback #21(u16 0) -> (w414:u16)
        n222 = Add(x=w412, y=w414) -> (x+y=w413:u16)
        "GI Late Counter 2" <- w413
        n223 = feedback-in #21(w413) -> ()
        n224 = feedback #22(i16 0) -> (w420:i16)
        n225 = Subtract(x=w420, y=w419) -> (x-y=w418:i16)
        "GI Relative phase 2" <- w418
        n226 = feedback-in #22(w418) -> ()
        n227 = feedback #23(TRUE) -> (w438:bool)
        n228 = case shown="2" "Operating Mode 2" {
          tunnel: [TRUE FALSE w463] -> w428
          tunnel: w438 -> [_ _ w460]
          frame 0, Default {
          }
          frame 1 {
          }
          frame 2 {
            n229 = Not(x=w460) -> (.not. x?=w462:bool)
            n230 = Select(t=w462, s="Invert GI 2", f=w460) -> (s? t:f=w463:bool)
          }
        }
        n231 = And(x=w428, y="Green FB On/Off") -> (x .and. y?=w407:bool)
        "green FB running" <- w407
        n232 = And(x=w407, y=w406) -> (x .and. y?=w405:bool)
        n233 = case shown="True" w405 {
          tunnel: "Current Out" -> [w447 _]
          tunnel: [w447 w452] -> w432
          frame False {
          }
          frame True {
            n234 = local read "Green FB Sum"() -> (w448:i16)
            n235 = call "Slower PID.vi"("process variable"=w448, "reset?"="Green FB Reset", "setpoint"="Green FB Setpoint", "PID gains (x 2^8)"="Green FB Gains", "output range"=cluster{"output high":i16, "output low":i16} {"output high"=32767, "output low"=-32768} ("Green FB output range")) -> ("output"=w456:i16)  [unwired: 10 out]
            n236 = To Long Integer(number=w456) -> (32bit integer=w449:i32)
            n237 = Add(x=w449, y=32768) -> (x+y=w451:i32)
            n238 = To Unsigned Word Integer(number=w451) -> (unsigned 16bit integer=w452:u16)
          }
        }
        n239 = Not(x=w438) -> (.not. x?=w435:bool)
        n240 = Select(t=w427, s=w435, f=w426) -> (s? t:f=w440:u32)
        n241 = Subtract(x=w440, y=w410) -> (x-y=w421:u32)
        n242 = Add(x=w421, y=w419) -> (x+y=w417:u32)
        n243 = feedback-in #23(w435) -> ()
        n244 = Boolean To (0,1)(Boolean=w428) -> (0, 1=w434:i16)
        n245 = To Unsigned Word Integer(number=w434) -> (unsigned 16bit integer=w431:u16)
        n246 = Multiply(x=w431, y=w432) -> (x*y=w433:u16)
      }
    }
  }
  n247 = while "APD 1 Counter" {
    tunnel: w4 -> [_]
    stop <- FALSE stop-if-true
    n248 = flat-sequence {
      frame #0 {
        n249 = xnode "FPGA I/O Method Node"("FPGA I/O In"=refnum<k21> "Connector0/DIO0" ("APD 1 DO"), "Timeout"=-1) -> ()  [unwired: 2 out]
      }
      frame #1 {
        n250 = local read "APD1 int gate"() -> (w467:bool)
        n251 = case shown="True" w467 {
          frame False {
          }
          frame True {
            n252 = local read "APD1 out state"() -> (w468:bool)
            n253 = case shown="True" w468 {
              frame False {
                n254 = local read "APD 1 Counts 0"() -> (w470:u32)
                n255 = Increment(x=w470) -> (x+1=→"APD 1 Counts 0":u32)
              }
              frame True {
                n256 = local read "APD 1 Counts 1"() -> (w472:u32)
                n257 = Increment(x=w472) -> (x+1=→"APD 1 Counts 1":u32)
              }
            }
          }
        }
      }
    }
  }
  n258 = while "RF synth board interlacing timing loop" {
    tunnel: w4 -> [_]
    stop <- FALSE stop-if-true
    # "This loop is stalled until the RF FIFO get a value. With this method we gain additional delay time (because  we allow the rest of the main RF loop to procede while this loop waits to send the switch signals - a form of parallelism). This helps to simplify the main RF code. \n\nThe code also allow optimal interlacing while also controlling trap RF phase. \n\nNote: a lot of work has gone into optimizing these methods and it is unclear how they can be made any faster or better than this (many failed tries). Right now there is essentially ~4 ticks (~90 ns ns) of imperfection in the switching from trap 1 to trap 2. ~2 ticks of no RF (phase reset) then ~2 ticks of trap 2 with the wrong amplitude (T1 amplitude). The total ticks is 200, so not a big error.\n\nPhase can be precisely set for each trap. Phase reset and switching, has similar delays as fsk frequency switching. And phase reset and phase offset changes are also not simultaneous. So we can't perfectly line everything up.\n\nIf you start from amp zero though (as for trap 1), the on switch is perfect. Likewise the off is perfect for trap 2. \n\nThe green laser switching is also perfect because of its reduced duty cycle and delays in fsk switching between 80 and 0 MHz."
    n259 = xnode ("FIFO Read")("Timeout"=-1) -> ("Element"=w519:u16, "FIFO Out"=w515:refnum<k21>)  [unwired: 1 in, 1 out]
    n260 = Equal To 0?(x=w519) -> (x = 0?=w516:bool)
    n261 = Not(x=w516) -> (.not. x?=w473:bool)
    n262 = flat-sequence "BD 1 and 2 RF phase and amplitude switching" {
      tunnel: w473 -> [_]
      tunnel: w508 -> [w623]
      tunnel: w507 -> [w622]
      tunnel: w506 -> [w621]
      tunnel: w505 -> [w620]
      tunnel: w504 -> [w619]
      tunnel: w503 -> [w618]
      tunnel: w502 -> [w617]
      tunnel: w501 -> [w616]
      tunnel: w499 -> [w615]
      tunnel: w498 -> [w614]
      tunnel: w497 -> [w613]
      tunnel: w495 -> [w611]
      tunnel: w494 -> [w610]
      tunnel: w493 -> [w609]
      tunnel: w496 -> [w612]
      tunnel: w500 -> [w608]
      tunnel: w492 -> [w647]
      tunnel: w491 -> [w646]
      tunnel: w490 -> [w645]
      tunnel: w489 -> [w644]
      tunnel: w488 -> [w643]
      tunnel: w487 -> [w642]
      tunnel: w486 -> [w641]
      tunnel: w485 -> [w640]
      tunnel: w484 -> [w639]
      tunnel: w482 -> [w638]
      tunnel: w481 -> [w637]
      tunnel: w480 -> [w636]
      tunnel: w479 -> [w635]
      tunnel: w478 -> [w634]
      tunnel: w477 -> [w633]
      tunnel: w483 -> [w632]
      frame #0 {
        # "Delay to align amp/frequency switching depending on the method used.\n\nCan also give enough time to do the parallel amplitude calculations"
        n263 = call "Wait2"("Count(Ticks)"="Amp switch delay") -> ()  [unwired: 1 out]
      }
      frame #1 {
        w603 = TRUE ("Connector1/DIO30")
        # "make phase offset and phase reset active with buffer transfer"
        n264 = xnode "FPGA I/O Node"("Connector1/DIO29"=w603, "Connector1/DIO30"=w603) -> ()  [unwired: 2 in, 2 out]
      }
      frame #2 {
        w604 = FALSE ("Connector1/DIO15")
        # "write phase restart to buffer and reset udclk"
        n265 = xnode "FPGA I/O Node"("Connector1/DIO29"=w604, "Connector1/DIO30"=w604, "Connector1/DIO15"=FALSE ("Connector1/DIO14")) -> ()  [unwired: 3 in, 3 out]
      }
      frame #3 {
        w606 = TRUE ("Connector1/DIO15")
        # "make phase restart active"
        # "reset WR"
        n266 = xnode "FPGA I/O Node"("Connector1/DIO15"=w606, "Connector1/DIO29"=w606, "Connector1/DIO30"=w606) -> ()  [unwired: 3 in, 3 out]
      }
      frame #4 {
        w607 = FALSE ("Connector1/DIO30")
        # "Address"
        # "set amp byte 1, and reset udclk"
        n267 = xnode "FPGA I/O Node"("Connector1/DIO0"=w623, "Connector1/DIO1"=w622, "Connector1/DIO2"=w621, "Connector1/DIO3"=w620, "Connector1/DIO4"=w619, "Connector1/DIO5"=w618, "Connector1/DIO6"=w617, "Connector1/DIO7"=w616, "Connector1/DIO8"=TRUE, "Connector1/DIO9"=FALSE, "Connector1/DIO10"=FALSE, "Connector1/DIO11"=FALSE, "Connector1/DIO12"=FALSE, "Connector1/DIO13"=TRUE, "Connector1/DIO20"=w608, "Connector1/DIO21"=w615, "Connector1/DIO22"=w614, "Connector1/DIO23"=w613, "Connector1/DIO24"=w612, "Connector1/DIO25"=w611, "Connector1/DIO26"=w610, "Connector1/DIO27"=w609, "Connector1/DIO30"=w607, "Connector1/DIO29"=w607) -> ()  [unwired: 24 in, 24 out]
      }
      frame #5 {
        # "write amp byte 1 to buffer"
        n268 = xnode "FPGA I/O Node"("Connector1/DIO15"=FALSE ("Connector1/DIO14")) -> ()  [unwired: 1 in, 1 out]
      }
      frame #6 {
        # "reset WR"
        n269 = xnode "FPGA I/O Node"("Connector1/DIO15"=TRUE) -> ()  [unwired: 1 in, 1 out]
      }
      frame #7 {
        # "Address"
        # "set amp byte 2"
        n270 = xnode "FPGA I/O Node"("Connector1/DIO0"=w647, "Connector1/DIO1"=w646, "Connector1/DIO2"=w645, "Connector1/DIO3"=w644, "Connector1/DIO4"=w643, "Connector1/DIO5"=w642, "Connector1/DIO6"=w641, "Connector1/DIO7"=w640, "Connector1/DIO8"=TRUE, "Connector1/DIO9"=FALSE, "Connector1/DIO10"=FALSE, "Connector1/DIO11"=FALSE, "Connector1/DIO12"=TRUE, "Connector1/DIO13"=FALSE, "Connector1/DIO20"=w639, "Connector1/DIO21"=w632, "Connector1/DIO22"=w638, "Connector1/DIO23"=w637, "Connector1/DIO24"=w636, "Connector1/DIO25"=w635, "Connector1/DIO26"=w634, "Connector1/DIO27"=w633) -> ()  [unwired: 22 in, 22 out]
      }
      frame #8 {
        # "write amp byte 2"
        n271 = xnode "FPGA I/O Node"("Connector1/DIO15"=FALSE ("Connector1/DIO14")) -> ()  [unwired: 1 in, 1 out]
      }
      frame #9 {
        w655 = TRUE ("Connector1/DIO15")
        # "transfer amp bytes 1 and 2 and reset WR"
        n272 = xnode "FPGA I/O Node"("Connector1/DIO29"=w655, "Connector1/DIO30"=w655, "Connector1/DIO15"=TRUE ("Connector1/DIO14")) -> ()  [unwired: 3 in, 3 out]
      }
      frame #10 {
        w657 = FALSE ("Connector1/DIO14")
        # "reset udclk"
        n273 = xnode "FPGA I/O Node"("Connector1/DIO29"=w657, "Connector1/DIO30"=w657) -> ()  [unwired: 2 in, 2 out]
      }
    }
    n274 = flat-sequence "FSK BD 1 (trap X)" {
      tunnel: w473 -> [w521]
      tunnel: [w521] -> w476
      tunnel: w476 -> [w522]
      frame #0 {
        n275 = call "Wait"("Count(Ticks)"="BD 1 Delay (ticks)") -> ()  [unwired: 1 out]
      }
      frame #1 {
        # "switch frequency"
        n276 = xnode "FPGA I/O Node"("Connector1/DIO36"=w522) -> ()  [unwired: 1 in, 1 out]
      }
    }
    n277 = flat-sequence "FSK BD 2 (trap Y or green laser AOM)" {
      tunnel: w473 -> [w659]
      tunnel: [w659] -> w518
      tunnel: w518 -> [w660]
      frame #0 {
        n278 = call "Wait3"("Count(Ticks)"="BD 2 Delay (Ticks)") -> ()  [unwired: 1 out]
      }
      frame #1 {
        # "switch frequency"
        n279 = xnode "FPGA I/O Node"("Connector1/DIO37"=w660) -> ()  [unwired: 1 in, 1 out]
      }
    }
    n280 = xnode ("FIFO Read")("Timeout"=-1, "FIFO In"=w515) -> ("Element"=w510:u16, "FIFO Out"=w514:refnum<k21>)  [unwired: 1 out]
    n281 = xnode ("FIFO Read")("Timeout"=-1, "FIFO In"=w514) -> ("Element"=w509:u16)  [unwired: 2 out]
    n282 = node-c288() -> (w512:T7)  [unwired: 1 in]
    n283 = timed-loop "Convert amplitude words to bits" {
      timing: w512 -> [_]
      timing-out: [_] -> w511
      tunnel: w510 -> [w579]
      tunnel: w509 -> [w578]
      tunnel: [w555] -> w508
      tunnel: [w554] -> w507
      tunnel: [w553] -> w506
      tunnel: [w552] -> w505
      tunnel: [w551] -> w504
      tunnel: [w550] -> w503
      tunnel: [w549] -> w502
      tunnel: [w548] -> w501
      tunnel: [w547] -> w500
      tunnel: [w546] -> w499
      tunnel: [w545] -> w498
      tunnel: [w544] -> w497
      tunnel: [w543] -> w496
      tunnel: [w542] -> w495
      tunnel: [w541] -> w494
      tunnel: [w540] -> w493
      tunnel: [w539] -> w492
      tunnel: [w538] -> w491
      tunnel: [w537] -> w490
      tunnel: [w536] -> w489
      tunnel: [w535] -> w488
      tunnel: [w534] -> w487
      tunnel: [w533] -> w486
      tunnel: [w532] -> w485
      tunnel: [w531] -> w484
      tunnel: [w530] -> w483
      tunnel: [w529] -> w482
      tunnel: [w528] -> w481
      tunnel: [w527] -> w480
      tunnel: [w526] -> w479
      tunnel: [w525] -> w478
      tunnel: [w524] -> w477
      stop <- TRUE stop-if-true
      # "Board 1 Data"
      # "Board 2 Data"
      # "Board 1 Data"
      # "Board 2 Data"
      n284 = Split Number(x=w579) -> (hi(x)=w577:u8, lo(x)=w557:u8)
      n285 = Split Number(x=w578) -> (hi(x)=w576:u8, lo(x)=w556:u8)
      n286 = Number To Boolean Array(number=w577) -> (Boolean array=w597:bool[])
      n287 = Number To Boolean Array(number=w576) -> (Boolean array=w588:bool[])
      n288 = Index Array(array=w597, index=7) -> (element=w555:bool)
      n289 = Index Array(array=w597, index=6) -> (element=w554:bool)
      n290 = Index Array(array=w597, index=5) -> (element=w553:bool)
      n291 = Index Array(array=w597, index=4) -> (element=w552:bool)
      n292 = Index Array(array=w597, index=3) -> (element=w551:bool)
      n293 = Index Array(array=w597, index=2) -> (element=w550:bool)
      n294 = Index Array(array=w597, index=1) -> (element=w549:bool)
      n295 = Index Array(array=w597, index=0) -> (element=w548:bool)
      n296 = Index Array(array=w588, index=7) -> (element=w547:bool)
      n297 = Index Array(array=w588, index=6) -> (element=w546:bool)
      n298 = Index Array(array=w588, index=5) -> (element=w545:bool)
      n299 = Index Array(array=w588, index=4) -> (element=w544:bool)
      n300 = Index Array(array=w588, index=3) -> (element=w543:bool)
      n301 = Index Array(array=w588, index=2) -> (element=w542:bool)
      n302 = Index Array(array=w588, index=1) -> (element=w541:bool)
      n303 = Index Array(array=w588, index=0) -> (element=w540:bool)
      n304 = Number To Boolean Array(number=w557) -> (Boolean array=w575:bool[])
      n305 = Number To Boolean Array(number=w556) -> (Boolean array=w566:bool[])
      n306 = Index Array(array=w575, index=7) -> (element=w539:bool)
      n307 = Index Array(array=w575, index=6) -> (element=w538:bool)
      n308 = Index Array(array=w575, index=5) -> (element=w537:bool)
      n309 = Index Array(array=w575, index=4) -> (element=w536:bool)
      n310 = Index Array(array=w575, index=3) -> (element=w535:bool)
      n311 = Index Array(array=w575, index=2) -> (element=w534:bool)
      n312 = Index Array(array=w575, index=1) -> (element=w533:bool)
      n313 = Index Array(array=w575, index=0) -> (element=w532:bool)
      n314 = Index Array(array=w566, index=7) -> (element=w531:bool)
      n315 = Index Array(array=w566, index=6) -> (element=w530:bool)
      n316 = Index Array(array=w566, index=5) -> (element=w529:bool)
      n317 = Index Array(array=w566, index=4) -> (element=w528:bool)
      n318 = Index Array(array=w566, index=3) -> (element=w527:bool)
      n319 = Index Array(array=w566, index=2) -> (element=w526:bool)
      n320 = Index Array(array=w566, index=1) -> (element=w525:bool)
      n321 = Index Array(array=w566, index=0) -> (element=w524:bool)
    }
    n322 = node-c288(w511) -> ()
  }
  n323 = while "APD 1 Gating" {
    shift-right: [w664] -> _
    shift-left: w4 -> [w669]
    shift-right: [w663] -> _
    shift-left: w6 -> [w661]
    stop <- FALSE stop-if-true
    n324 = flat-sequence {
      tunnel: w669 -> [w672]
      tunnel: [w673] -> w667
      tunnel: [w672] -> w665
      tunnel: [w671] -> w662
      tunnel: w661 -> [w671]
      tunnel: [w676] -> w668
      tunnel: w667 -> [w676]
      tunnel: [w675] -> w666
      tunnel: w665 -> [w675]
      tunnel: w662 -> [w674]
      tunnel: [w696] -> w664
      tunnel: w668 -> [w710]
      tunnel: w666 -> [w707]
      tunnel: [w678] -> w663
      frame #0 {
        n325 = call "Loop Timer4"("Count(Ticks)"=w672) -> ("Tick Count(Ticks)"=w673:u32)
      }
      frame #1 {
        # "Signal maybe then sent through \na transistor before APD"
        n326 = xnode "FPGA I/O Node"("Connector1/DIO33"=w674) -> ()  [unwired: 1 in, 1 out]
        "APD1 int gate" <- w674
      }
      frame #2 {
        n327 = feedback #24(TRUE) -> (w702:bool)
        n328 = feedback-in #25(w710) -> ()
        n329 = feedback #25(w710) -> (w709:u32)
        n330 = Not(x=w702) -> (.not. x?=w699:bool)
        n331 = feedback-in #24(w699) -> ()
        n332 = Subtract(x=w710, y=w709) -> (x-y=w708:u32)
        n333 = Select(t="APD Gate ON Count", s=w699, f="APD Gate OFF Count") -> (s? t:f=w704:u16)
        n334 = Subtract(x=w708, y=w707) -> (x-y=w684:u32)
        n335 = Subtract(x=w704, y=w684) -> (x-y=w695:u32)
        n336 = Number To Boolean Array(number=w684) -> (Boolean array=w685:bool[])
        n337 = Or Array Elements(Boolean array=w685) -> (logical OR=w683:bool)
        n338 = Boolean To (0,1)(Boolean="+ phase (APD 1 Gate)") -> (0, 1=w693:i16)
        n339 = Boolean To (0,1)(Boolean=w683) -> (0, 1=w690:i16)
        n340 = Multiply(x=w693, y="Phase count adjustment (APD 1 Gate)") -> (x*y=w691:i16)
        n341 = To Unsigned Byte Integer(number=w690) -> (unsigned 8bit integer=w687:u8)
        n342 = Add(x=w695, y=w691) -> (x+y=w696:u32)
        n343 = feedback #26(i16 0) -> (w698:i16)
        n344 = Subtract(x=w698, y=w691) -> (x-y=w697:i16)
        "APD 1 Gate Relative Phase" <- w697
        n345 = feedback-in #26(w697) -> ()
        n346 = feedback #27(u8 0) -> (w688:u8)
        n347 = Add(x=w687, y=w688) -> (x+y=w686:u8)
        "APD 1 Gate Late Counter" <- w686
        n348 = feedback-in #27(w686) -> ()
        n349 = local read "Green long-scale interlacing"() -> (w677:bool)
        n350 = case shown="2" "APD Gate Operating Mode" {
          tunnel: [TRUE FALSE w732] -> w680
          tunnel: w702 -> [_ _ w732]
          frame 0, Default {
          }
          frame 1 {
          }
          frame 2 {
          }
        }
        n351 = Not(x=w680) -> (.not. x?=w681:bool)
        n352 = Select(t=w681, s="Invert APD Gate", f=w680) -> (s? t:f=w679:bool)
        n353 = case shown="True" w677 {
          tunnel: w679 -> [w711 w719]
          tunnel: [w711 w720] -> w678
          frame False {
          }
          frame True {
            n354 = local read "Number of ON cycles"() -> (w713:i16)
            n355 = local read "Number of OFF cycles"() -> (w715:i16)
            n356 = feedback #28(i16 1) -> (w726:i16)
            n357 = Increment(x=w726) -> (x+1=w725:i16)
            n358 = feedback #29(w713) -> (w712:i16)
            n359 = Greater?(x=w712, y=w726) -> (0:w721:bool)
            n360 = Select(t=w725, s=w721, f=i16 1) -> (s? t:f=w723:i16)
            n361 = feedback-in #28(w723) -> ()
            n362 = feedback #30(TRUE) -> (w718:bool)
            n363 = Not(x=w718) -> (.not. x?=w717:bool)
            n364 = Select(t=w718, s=w721, f=w717) -> (s? t:f=w716:bool)
            n365 = feedback-in #30(w716) -> ()
            n366 = Select(t=w713, s=w716, f=w715) -> (s? t:f=w714:i16)
            n367 = feedback-in #29(w714) -> ()
            n368 = case shown="True" w716 {
              tunnel: [FALSE w729] -> w720
              tunnel: w719 -> [_ w729]
              frame False {
              }
              frame True {
              }
            }
          }
        }
      }
    }
  }
  n369 = while "Trap RF control, main calculations (raster scanning, intensity and position feedback, phase control etc) with primary timing trigger" {
    shift-right: [w751] -> _
    shift-left: w4 -> [w750]
    shift-right: [w749] -> _
    shift-left: FALSE ("Swap F1 and F2") -> [w748]
    shift-right: [w744] -> _
    shift-left: u16 0 ("BD 1 Amplitude 3") -> [w741]
    shift-right: [w743] -> _
    shift-left: u16 0 ("BD 2 Amplitude 3") -> [w739]
    shift-right: [w738] -> _
    shift-left: u64 0 -> [w737]
    shift-right: [w736] -> _
    shift-left: i64 0 -> [w735]
    shift-right: [w734] -> _
    shift-left: i64 0 -> [w733]
    stop <- FALSE stop-if-true
    n370 = flat-sequence {
      tunnel: w748 -> [w757]
      tunnel: w750 -> [w754]
      tunnel: [w757] -> w747
      tunnel: [w753] -> w746
      tunnel: [w754] -> w745
      tunnel: [w756] -> w742
      tunnel: w741 -> [w756]
      tunnel: [w755] -> w740
      tunnel: w739 -> [w755]
      tunnel: [w772] -> w751
      tunnel: [w771] -> w749
      tunnel: w747 -> [w770]
      tunnel: w746 -> [w769]
      tunnel: w745 -> [w768]
      tunnel: [w767] -> w744
      tunnel: [w766] -> w743
      tunnel: w742 -> [w765]
      tunnel: w740 -> [w764]
      tunnel: [w763] -> w738
      tunnel: w737 -> [w762]
      tunnel: [w761] -> w736
      tunnel: w735 -> [w760]
      tunnel: [w759] -> w734
      tunnel: w733 -> [w758]
      frame #0 {
        n371 = call "Loop Timer2"("Count(Ticks)"=w754) -> ("Tick Count(Ticks)"=w753:u32)
      }
      frame #1 {
        n372 = flat-sequence {
          tunnel: w770 -> [w780]
          tunnel: w765 -> [w774]
          tunnel: w764 -> [w773]
          tunnel: [w844] -> w772
          tunnel: [w856] -> w771
          tunnel: w769 -> [w850]
          tunnel: w768 -> [w847]
          tunnel: [w795] -> w767
          tunnel: [w794] -> w766
          tunnel: [w786] -> w763
          tunnel: w762 -> [w785]
          tunnel: [w784] -> w761
          tunnel: w760 -> [w783]
          tunnel: [w782] -> w759
          tunnel: w758 -> [w781]
          frame #0 {
            w775 = -1 ("Timeout")
            # "Operation when you need a long delay for either X or Y to synchonize AOD light out phase (> ~100 ticks)\nor want shorter trap ON timing. Puts some of the delay timing in parallel with the later computations."
            # "Trigger the external loop by sending the boolean FSK value through a FIFO.\nTiming is precise."
            n373 = Boolean To (0,1)(Boolean=w780) -> (0, 1=w779:i16)
            n374 = To Unsigned Word Integer(number=w779) -> (unsigned 16bit integer=w778:u16)
            n375 = xnode ("FIFO Method Node")("Element"=w778, "Timeout"=w775) -> ("FIFO Out"=w777:refnum<k21>)  [unwired: 1 in, 1 out]
            n376 = xnode ("FIFO Method Node")("Element"=w774, "Timeout"=w775, "FIFO In"=w777) -> ("FIFO Out"=w776:refnum<k21>)  [unwired: 1 out]
            n377 = xnode ("FIFO Method Node")("Element"=w773, "Timeout"=w775, "FIFO In"=w776) -> ()  [unwired: 2 out]
          }
          frame #1 {
            # "Just counts, wraps around, 8 bit"
            # "Which trap cycle"
            # "Only save the 3rd set's amp in the loop"
            # "If this is NOT set 3 AND NOT (RF synth controls green AND green FB running)\nthen use this sets amp value (otherwise keep the green feedback value)"
            # "Just flips back and forth."
            # "If interlacing is off, this is which cycle to use."
            # "Keep track of trap cycles (trap 1, 2, 3...)"
            # "This is the prior cycle's on time"
            # "increment timing\nindex, reset to 0 if \nend of matrix"
            # "Reset to begginning (1) when number of cycles reached."
            # "timing index"
            # "build byte stacks for writing data\n(must correspond to addresses array constant)"
            # "Timing housekeeping"
            # "Adjust phase if late\n(maintains constant phase relationship between cycles)"
            n378 = feedback #31(u8 0 ("t")) -> (w853:u8)
            n379 = Increment(x=w853) -> (x+1=w892:u8)
            n380 = Increment(x="Number Interlace Cycles") -> (x+1=w887:u8)
            n381 = Equal?(x=w892, y=w887) -> (x = y?=w894:bool)
            n382 = Select(t=u8 1, s=w894, f=w892) -> (s? t:f=w852:u8)
            n383 = feedback-in #31(w852) -> ()
            n384 = Increment(x=w852) -> (x+1=w889:u8)
            n385 = Equal?(x=w889, y=w887) -> (x = y?=w890:bool)
            n386 = Select "This cycle"(t=u8 1, s=w890, f=w889) -> (s? t:f=w886:u8)
            n387 = Select(t=w886, s="Interlace ON/OFF", f="Interlace Off Parameters") -> (s? t:f=w805:u8)
            n388 = feedback-in #32(w850) -> ()
            n389 = feedback #32(w850) -> (w849:u32)
            n390 = Select(t=w852, s="Interlace ON/OFF", f="Interlace Off Parameters") -> (s? t:f=w885:u8)
            n391 = Subtract(x=w850, y=w849) -> (x-y=w848:u32)
            n392 = Subtract "The error"(x=w848, y=w847) -> (x-y=w831:u32)
            n393 = case shown="1, Default" w885 {
              tunnel: ["DIO count 1 (ticks)" "DIO count 2 (ticks)" "DIO count 3 (ticks)"] -> w846
              frame 1, Default {
              }
              frame 2 {
              }
              frame 3 {
              }
            }
            n394 = Number To Boolean Array(number=w831) -> (Boolean array=w832:bool[])
            n395 = Or Array Elements(Boolean array=w832) -> (logical OR=w830:bool)
            n396 = Boolean To (0,1)(Boolean=w830) -> (0, 1=w837:i16)
            n397 = To Unsigned Byte Integer(number=w837) -> (unsigned 8bit integer=w834:u8)
            n398 = feedback #33(u8 0) -> (w835:u8)
            n399 = Add(x=w834, y=w835) -> (x+y=w833:u8)
            "DIO Late Counter" <- w833
            n400 = feedback-in #33(w833) -> ()
            n401 = Subtract(x=w846, y=w831) -> (x-y=w845:u32)
            n402 = disable-structure shown="Disabled" {
              disable-tunnel: [w898 _] -> w829
              disable-tunnel: w805 -> [w895 _]
              frame Disabled {
                n403 = feedback #34(i64 0 ("y")) -> (w897:i64)
                n404 = case "Synchronize trap oscillations - always begin/end with trap 1" shown="1, Default" w895 {
                  tunnel: [w899 w900 w901] -> w898
                  tunnel: w897 -> [w899 w900 _]
                  frame 2 {
                  }
                  frame 3 {
                  }
                  frame 1, Default {
                    n405 = Or(x="Osc traps", y="Initiate trap osc") -> (x .or. y?=w903:bool)
                    n406 = case "Trap sine oscillation (or whatever pattern is stored in memory)" shown="True" w903 {
                      tunnel: [i64 0 ("y") w907] -> w901
                      tunnel: "Initiate trap osc" -> [_ w910]
                      frame False {
                      }
                      frame True {
                        w914 = u16 0
                        w912 = -1
                        n407 = local write "Initiate trap osc"(FALSE ("Initiate trap osc")) -> ()
                        n408 = feedback #35(w914) -> (w916:u16)
                        n409 = Select(t=w914, s=w910, f=w916) -> (s? t:f=w915:u16)
                        n410 = Greater Or Equal?(x=w915, y="Trap osc period (pts)") -> (x >= y?=w921:bool)
                        n411 = Or(x=w910, y=w921) -> (x .or. y?=w922:bool)
                        n412 = Select(t=u16 0, s=w922, f=w915) -> (s? t:f=w906:u16)
                        n413 = feedback #36(w912) -> (w913:i32)
                        n414 = Select(t=w912, s=w910, f=w913) -> (s? t:f=w911:i32)
                        n415 = Increment(x=w911) -> (x+1=w918:i32)
                        n416 = Equal?(x=w906, y=u16 0) -> (x = y?=w919:bool)
                        n417 = Increment(x=w906) -> (x+1=w926:u16)
                        n418 = feedback-in #35(w926) -> ()
                        n419 = Select(t=w918, s=w919, f=w911) -> (s? t:f=w917:i32)
                        n420 = feedback-in #36(w917) -> ()
                        n421 = case shown="False" "Osc trap cont." {
                          tunnel: w917 -> [w930 _]
                          frame False {
                            n422 = Greater Or Equal?(x=w930, y="N trap osc periods") -> (x >= y?=w928:bool)
                            n423 = Not(x=w928) -> (.not. x?=w927:bool)
                            n424 = local write "Osc traps"(w927) -> ()
                          }
                          frame True {
                          }
                        }
                        n425 = xnode ("Memory Read")("Address"=w906, "Memory In"=refnum<k21> "Trap osc memory") -> ("Data"=w907:i64)  [unwired: 1 out]
                      }
                    }
                  }
                }
                n426 = feedback-in #34(w898) -> ()
              }
              frame Enabled {
              }
            }
            n427 = local read "green FB running"() -> (w818:bool)
            n428 = And(x=w818, y="RF synth bd controls green") -> (x .and. y?=w817:bool)
            n429 = case shown="1, Default" w805 {
              tunnel: [w1061 w1311 "BD 1 Frequency 3"] -> w882
              tunnel: [w1101 w1310 w1339] -> w821
              tunnel: ["BD 2 Amplitude 1" "BD 2 Amplitude 2" w1338] -> w813
              tunnel: [w1058 w1307 "BD 1 Amplitude 3"] -> w795
              tunnel: "FB Gains" -> [w1078 w1317 _]
              tunnel: "FB output range" -> [w1079 w1316 _]
              tunnel: w829 -> [w1076 w1314 _]
              tunnel: "BD 2 Frequency 1" -> [w1073 _ _]
              tunnel: "BD 2 Frequency 2" -> [_ w1310 _]
              tunnel: "BD 2 Frequency 3" -> [_ _ w1339]
              tunnel: w817 -> [_ _ w1337]
              tunnel: [w1061 w1308 w1336] -> w786
              tunnel: w785 -> [w1060 w1308 w1336]
              tunnel: [w1047 i64 0 i64 0] -> w784
              tunnel: w783 -> [_ w1303 _]
              tunnel: [w1046 i64 0 i64 0] -> w782
              tunnel: w781 -> [_ w1301 _]
              frame 1, Default {
                w1092 = fxp<+/-,24,9> 0.0 ("AI1 X Set 2")
                w1086 = u16 0
                w1099 = i64 0 ("f")
                # "Changed by Ronen - correction \nby PID is now implemented not on \nthe Base BD1 frequency but on the last\nfrequency sent."
                # "Added by Ronen -\nUpper and Lower \nLimits for the FB \ngenerated frequency\nto avoid losing bead \nwhen tether breaks"
                # "Explanation of raster scanning:\n1. Cycles: increment counter by 1 every time interlace cycle returns to trap 1. As long as \n  Cycle per Step is larger than counter, keep incrementing counter and do not change step counter.\n  Once counter is equal to Cycles per step, zero counter and increment step counter.\n2. Steps: Increments up every time cycles counter equals cycles per step. Performs the following:\n- To determine DIRECTION of frequency change:  If ScanstepX2 is EQUAL to step counter (full for-back scan finished)\n   frequency increment is set to zero, AND step counter is set to zero. \n   Otherwise: if no change to step counter (because cycleperstep>cycle counter), then no change to frequency\n   increment. \n   If step counter has changed (cycleperstep=cycle counter), then need to figure out direction of frequency change:\n   if step counter is EQUAL to Scansteps: No change to frequency increment\n   Otherwise: If scan steps > step counter - 1 (forward scan NOT completed): increment frequency by 1\n                       If scan steps equal or smaller than step counter -1 (forward scan completed): increment frequency by -1\n\n3. Scans: Increment scan counter every time step counter equals 2Xscan steps (full for-back scan completed)\n    if number of scans > scan counter: Send TRUE to scanning, continue scan\n    if number of scans = scan counter: Send FALSE to Scanning, Scan finished.\n\n  The wire with the asterik can be used as the index for getting the mirror positions in the offset scan."
                # "This signal integration happens no matter what\nso that correct setpoints can be chosen before \nturning on the FB."
                # "Trap 1"
                n430 = local read "AI1 X Set 2"() -> (w1071:fxp<+/-,16,1>)
                n431 = local read "AI1 X Set 1"() -> (w1089:fxp<+/-,16,1>)
                n432 = local read "Scanning"() -> (w1102:bool)
                n433 = Multiply(x=w1071, y="B factor") -> (x*y=w1069:fxp<+/-,48,17>)
                n434 = Or(x=w1102, y="Start scan") -> (x .or. y?=w1056:bool)
                n435 = case shown="True" "Diff FB Measurement?" {
                  tunnel: w1069 -> [w1200 w1209]
                  tunnel: w1089 -> [w1199 w1210]
                  tunnel: [w1197 w1201] -> w1090
                  frame False {
                    n436 = Select(t=w1199, s="Trap Pos FB Monitor T1 or T2", f=w1200) -> (s? t:f=w1197:fxp<+/-,48,17>)
                  }
                  frame True {
                    n437 = Subtract(x=w1210, y=w1209) -> (x-y=w1202:fxp<+/-,48,17>)
                    n438 = Not(x="Negate Diff?") -> (.not. x?=w1208:bool)
                    n439 = Boolean To (0,1)(Boolean="Negate Diff?") -> (0, 1=w1206:i16)
                    n440 = Boolean To (0,1)(Boolean=w1208) -> (0, 1=w1207:i16)
                    n441 = Negate(x=w1206) -> (-x=w1205:i16)
                    n442 = Add(x=w1205, y=w1207) -> (x+y=w1203:i16)
                    n443 = Multiply(x=w1203, y=w1202) -> (x*y=w1201:fxp<+/-,63,32>)
                  }
                }
                n444 = feedback #37(w1086) -> (w1085:u16)
                n445 = Increment(x=w1085) -> (x+1=w1087:u16)
                n446 = Greater Or Equal?(x=w1087, y="Trap Pos FB Int Count") -> (x >= y?=w1059:bool)
                n447 = Select(t=w1086, s=w1059, f=w1087) -> (s? t:f=w1088:u16)
                n448 = feedback-in #37(w1088) -> ()
                n449 = feedback #38(w1092) -> (w1091:fxp<+/-,24,9>)
                n450 = Add(x=w1090, y=w1091) -> (x+y=w1084:fxp<+/-,24,9>)
                n451 = Select(t=w1092, s=w1059, f=w1084) -> (s? t:f=w1095:fxp<+/-,24,9>)
                n452 = feedback-in #38(w1095) -> ()
                n453 = case "Trap 1 X intensity feedback" shown="True" "FB On/Off Set 1" {
                  tunnel: "BD 1 Amplitude 1" -> [w1292 _]
                  tunnel: [w1292 w1296] -> w1058
                  tunnel: w1079 -> [_ w1293]
                  tunnel: w1078 -> [_ w1294]
                  frame False {
                  }
                  frame True {
                    n454 = local read "AI2 Y Sum Set 1"() -> (w1297:i16)
                    n455 = call "Slower PID.vi"("process variable"=w1297, "reset?"="FB Reset Set 1", "setpoint"="FB Setpoint Set 1", "PID gains (x 2^8)"=w1294, "output range"=w1293) -> ("output"=w1298:i16)  [unwired: 10 out]
                    n456 = To Unsigned Word Integer(number=w1298) -> (unsigned 16bit integer=w1296:u16)
                  }
                }
                "BD1 amplitude 1 out" <- w1058
                n457 = Divide(x=w1084, y="Trap Pos FB Int Count") -> (x/y=w1057:fxp<+/-,16,1>)
                n458 = case "For raster scanning" shown="True" w1056 {
                  tunnel: [i64 0 w1140] -> w1048
                  tunnel: [FALSE w1128] -> w1051
                  tunnel: [i16 0 w1127] -> w1052
                  tunnel: w1057 -> [_ w1126]
                  tunnel: "Start scan" -> [_ w1120]
                  frame False {
                    n459 = local write "Scanning"(FALSE ("scanning")) -> ()
                  }
                  frame True {
                    w1134 = u64 0
                    # "Changed by RG, to introduce force\ndependent stopping of the raster scan \nand manual stopping"
                    # "count number of cycles"
                    n460 = feedback #39(w1134) -> (w1137:u64)
                    n461 = Select(t=w1134, s=w1120, f=w1137) -> (s? t:f=w1139:u64)
                    n462 = Increment(x=w1139) -> (x+1=w1132:u64)
                    n463 = Equal?(x=i16 1, y=w1132) -> (x = y?=w1130:bool)
                    n464 = And(x="Abort scan", y=w1130) -> (x .and. y?=w1128:bool)
                    n465 = Greater?(x="Cycles per step", y=w1132) -> (0:w1135:bool)
                    n466 = Select(t=w1132, s=w1135, f=w1134) -> (s? t:f=w1136:u64)
                    n467 = feedback-in #39(w1136) -> ()
                    n468 = Greater?(x=w1126, y="Raster setpoint") -> (0:w1123:bool)
                    n469 = And(x=w1123, y="Raster to target force") -> (x .and. y?=w1121:bool)
                    n470 = case shown="False" w1128 {
                      tunnel: [w1147 i16 0] -> w1140
                      tunnel: w1120 -> [w1172 _]
                      tunnel: w1135 -> [w1165 _]
                      tunnel: w1134 -> [w1155 _]
                      tunnel: [w1149 FALSE] -> w1129
                      tunnel: [w1145 w1183] -> w1127
                      tunnel: [w1148 w1184] -> w1124
                      frame False {
                        w1156 = i64 0
                        # "scan incr."
                        # "freq. incr. mult."
                        # "count steps"
                        n471 = feedback #40(w1155) -> (w1180:u64)
                        n472 = Select(t=w1155, s=w1172, f=w1180) -> (s? t:f=w1148:u64)
                        n473 = Increment(x=w1148) -> (x+1=w1179:u64)
                        n474 = Add(x="Scan steps", y="Scan steps") -> (x+y=w1178:u64)
                        n475 = Select(t=w1148, s=w1165, f=w1179) -> (s? t:f=w1160:u64)
                        n476 = Greater?(x=w1178, y=w1160) -> (0:w1159:bool)
                        n477 = Select(t=w1160, s=w1159, f=w1155) -> (s? t:f=w1176:u64)
                        n478 = feedback-in #40(w1176) -> ()
                        n479 = Equal?(x="Scan steps", y=w1160) -> (x = y?=w1164:bool)
                        n480 = Greater?(x="Scan steps", y=w1148) -> (0:w1175:bool)
                        n481 = feedback #41(w1156) -> (w1177:i64)
                        n482 = Select(t=w1156, s=w1172, f=w1177) -> (s? t:f=w1162:i64)
                        n483 = Increment(x=w1162) -> (x+1=w1174:i64)
                        n484 = Decrement(x=w1162) -> (x-1=w1173:i64)
                        n485 = Select(t=w1174, s=w1175, f=w1173) -> (s? t:f=w1163:i64)
                        n486 = Select(t=w1162, s=w1164, f=w1163) -> (s? t:f=w1161:i64)
                        n487 = Select(t=w1162, s=w1165, f=w1161) -> (s? t:f=w1157:i64)
                        n488 = Select(t=w1157, s=w1159, f=w1156) -> (s? t:f=w1158:i64)
                        n489 = feedback-in #41(w1158) -> ()
                        n490 = feedback #42(w1155) -> (w1171:u64)
                        n491 = Select(t=w1155, s=w1172, f=w1171) -> (s? t:f=w1167:u64)
                        n492 = Increment(x=w1167) -> (x+1=w1168:u64)
                        n493 = Select(t=w1167, s=w1159, f=w1168) -> (s? t:f=w1166:u64)
                        n494 = Greater?(x="Number of scans", y=w1166) -> (0:w1152:bool)
                        n495 = Multiply(x="Scan freq.  increment", y=w1162) -> (x*y=w1147:i64)
                        n496 = Select(t=TRUE, s="Cont. Scan", f=w1152) -> (s? t:f=w1149:bool)
                        n497 = Select(t=w1166, s=w1149, f=w1155) -> (s? t:f=w1169:u64)
                        n498 = feedback-in #42(w1169) -> ()
                        n499 = local read "BD 1 Frequency 1"() -> (w1146:u64)
                        n500 = Increment(x=w1166) -> (x+1=→"Scan I":u64)
                        n501 = Add(x=w1147, y=w1146) -> (x+y=w1145:u64)
                        "Actual Scan freq" <- w1145
                      }
                      frame True {
                        n502 = local read "Actual Scan freq"() -> (w1183:u64)
                        n503 = local read "Scan steps"() -> (w1184:u64)
                      }
                    }
                    "Scanning" <- w1129
                    n504 = case shown="True" w1121 {
                      tunnel: w1124 -> [_ w1144]
                      frame False {
                      }
                      frame True {
                        n505 = Add(x=w1144, y=i16 2) -> (x+y=w1142:u64)
                        n506 = local write "Raster to target force"(FALSE) -> ()
                        n507 = local write "Scan steps"(w1142) -> ()
                      }
                    }
                  }
                }
                n508 = feedback #43(fxp<+/-,24,9> 0.0 ("AI1 X Set 2")) -> (w1096:fxp<+/-,24,9>)
                n509 = Select(t=w1084, s=w1059, f=w1096) -> (s? t:f=w1097:fxp<+/-,24,9>)
                "Trap Pos FB Int Signal" <- w1097
                n510 = feedback-in #43(w1097) -> ()
                n511 = feedback #44(fxp<+/-,16,1> 0.0 ("Trap Pos FB Int-Norm Signal")) -> (w1081:fxp<+/-,16,1>)
                n512 = Select(t=w1057, s=w1059, f=w1081) -> (s? t:f=w1080:fxp<+/-,16,1>)
                "Trap Pos FB Int-Norm Signal" <- w1080
                n513 = feedback-in #44(w1080) -> ()
                n514 = case "For position feedback" shown="True" "Force feedback" {
                  tunnel: [i64 0 w1216] -> w1049
                  tunnel: w1057 -> [_ w1213]
                  tunnel: w1059 -> [_ w1212]
                  frame False {
                  }
                  frame True {
                    n515 = feedback #45(i64 0) -> (w1215:i64)
                    n516 = case shown="True" w1212 {
                      tunnel: [w1217 w1221] -> w1216
                      tunnel: w1215 -> [w1217 _]
                      tunnel: w1213 -> [_ w1220]
                      frame False {
                      }
                      frame True {
                        n517 = xnode ("PID")("process variable"=w1220, "reset?"="Trap Pos. FB Reset", "setpoint"="Trap Pos. FB SP", "PID gains"="Trap Pos. FB Gains", "output range"="Trap pos. FB Range") -> ("output"=w1230:fxp<+/-,16,1>)
                        n518 = Negate(x=w1230) -> (-x=w1229:fxp<+/-,17,2>)
                        n519 = Select(t=w1229, s="Trap Pos FB Negate Action", f=w1230) -> (s? t:f=w1226:fxp<+/-,17,2>)
                        n520 = Scale By Power Of 2(n=u32 15, x=u32 1) -> (x*2^n=w1223:u32)
                        n521 = Multiply(x=w1226, y=w1223) -> (x*y=w1222:fxp<+/-,17,17>)
                        n522 = To Quad Integer(1:w1222) -> (0:w1234:i64)
                        "Trap Pos FB Action" <- w1234
                        n523 = Multiply(x=w1234, y="Trap Pos. FB Mult Factor") -> (x*y=w1232:i64)
                        n524 = Add(x=w1232, y="Trap Pos. FB Offset Factor") -> (x+y=w1221:i64)
                        n525 = disable-structure shown="Disabled" {
                          disable-tunnel: w1221 -> [w1241 _]
                          frame Disabled {
                            w1245 = u32 0
                            n526 = feedback #46() -> (w1242:i64)  [unwired: 1 in]
                            n527 = Add(x=w1241, y=w1242) -> (x+y=w1239:i64)
                            n528 = feedback #47(w1245) -> (w1247:u32)
                            n529 = Increment(x=w1247) -> (x+1=w1236:u32)
                            n530 = Greater Or Equal?(x=w1236, y="FB Trig Integrate") -> (x >= y?=w1237:bool)
                            n531 = Select(t=i64 0, s=w1237, f=w1239) -> (s? t:f=w1243:i64)
                            n532 = feedback-in #46(w1243) -> ()
                            n533 = Select(t=w1245, s=w1237, f=w1236) -> (s? t:f=w1246:u32)
                            n534 = feedback-in #47(w1246) -> ()
                            n535 = And(x=w1237, y="FPGA Trap Trig") -> (x .and. y?=w1244:bool)
                            n536 = case "Trap FB trigger excitation laser ON" shown="True" w1244 {
                              tunnel: w1239 -> [_ w1251]
                              tunnel: w1236 -> [_ w1249]
                              frame False {
                              }
                              frame True {
                                n537 = Not(x="TTrig Negate Pos") -> (.not. x?=w1258:bool)
                                n538 = Boolean To (0,1)(Boolean="TTrig Negate Pos") -> (0, 1=w1256:i16)
                                n539 = Boolean To (0,1)(Boolean=w1258) -> (0, 1=w1257:i16)
                                n540 = Negate(x=w1256) -> (-x=w1255:i16)
                                n541 = Add(x=w1255, y=w1257) -> (x+y=w1254:i16)
                                n542 = Multiply(x=w1254, y=w1251) -> (x*y=w1253:i64)
                                "TTrig Sig" <- w1253
                                n543 = Multiply(x="FPGA TTrig Thresh", y=w1249) -> (x*y=w1250:i64)
                                "TTrig Fin Thresh" <- w1250
                                n544 = Greater Or Equal?(x=w1253, y=w1250) -> (x >= y?=w1252:bool)
                                n545 = case shown="True" w1252 {
                                frame False {
                                }
                                frame True {
                                w1261 = TRUE ("Green FB On/Off")
                                w1263 = u8 2 ("Operating Mode")
                                n546 = local write "Operating Mode"(w1263) -> ()
                                n547 = local write item#-1(w1263) -> ()
                                n548 = local write item#-1(w1261) -> ()
                                n549 = local write "FPGA Trap Trig"(FALSE ("FPGA Trap Trig")) -> ()
                                "TTrig?" <- w1261
                                }
                                }
                              }
                            }
                          }
                          frame Enabled {
                          }
                        }
                      }
                    }
                    n550 = feedback-in #45(w1216) -> ()
                  }
                }
                n551 = case shown="True" "Symmetric FB/Raster" {
                  tunnel: [w1106 w1110] -> w1046
                  tunnel: w1049 -> [w1106 w1111]
                  tunnel: w1048 -> [w1105 w1108]
                  tunnel: [w1105 w1107] -> w1047
                  frame False {
                  }
                  frame True {
                    n552 = Scale By Power Of 2(n=i16 -1, x=w1111) -> (x*2^n=w1110:i64)
                    n553 = Scale By Power Of 2(n=i16 -1, x=w1108) -> (x*2^n=w1107:i64)
                  }
                }
                n554 = And(x="Force feedback", y="Dynamic Force FB (Ronen)") -> (x .and. y?=w1066:bool)
                n555 = case shown="False" w1066 {
                  tunnel: w1046 -> [w1188 w1192]
                  tunnel: [w1187 w1191] -> w1053
                  tunnel: w1060 -> [_ w1190]
                  tunnel: w1059 -> [_ w1189]
                  frame False {
                    # "(BD1 Frequency 1)"
                    n556 = Add(x="BD 1 Frequency 1", y=w1188) -> (x+y=w1187:u64)
                  }
                  frame True {
                    n557 = case shown="True" w1189 {
                      tunnel: w1192 -> [_ w1196]
                      tunnel: [w1193 w1195] -> w1191
                      tunnel: w1190 -> [w1193 w1194]
                      frame False {
                      }
                      frame True {
                        n558 = Add(x=w1194, y=w1196) -> (x+y=w1195:u64)
                      }
                    }
                  }
                }
                n559 = case shown="False" w1051 {
                  tunnel: [w1113 w1115] -> w1054
                  tunnel: w1053 -> [w1113 _]
                  tunnel: w1052 -> [_ w1115]
                  frame False {
                  }
                  frame True {
                    n560 = local write "BD 1 Frequency 1"(w1115) -> ()
                    n561 = local write "Abort scan"(FALSE) -> ()
                  }
                }
                n562 = Select(t=w1076, s="Trap 1 osc enable", f=i64 0) -> (s? t:f=w1074:i64)
                n563 = Select(t=w1099, s="Scan BD", f=w1047) -> (s? t:f=w1098:i64)
                n564 = Select(t=w1047, s="Scan BD", f=w1099) -> (s? t:f=w1065:i64)
                n565 = Add(x=w1098, y=w1073) -> (x+y=w1101:u64)
                n566 = Compound Arithmetic op=ADD(w1074, w1054, w1065) -> (w1064:u64)
                n567 = In Range and Coerce(upper limit="FB Max Frequency", x=w1064, lower limit="FB Min frequency") -> (coerced(x)=w1061:u64)  [unwired: 1 out]
                "BD1 Frequency Out 1" <- w1061
              }
              frame 2 {
                # "Trap 2"
                n568 = local read "Symmetric FB/Raster"() -> (w1306:bool)
                n569 = case shown="True" w1306 {
                  tunnel: "BD 1 Frequency 2" -> [w1320 w1325]
                  tunnel: [w1320 w1321] -> w1304
                  tunnel: w1303 -> [_ w1324]
                  tunnel: w1301 -> [_ w1323]
                  frame False {
                  }
                  frame True {
                    n570 = Subtract(x=w1325, y=w1324) -> (x-y=w1322:u64)
                    n571 = Subtract(x=w1322, y=w1323) -> (x-y=w1321:u64)
                  }
                }
                n572 = case "Trap 2 X intensity feedback" shown="True" "FB On/Off Set 2" {
                  tunnel: [w1326 w1329] -> w1307
                  tunnel: "BD 1 Amplitude 2" -> [w1326 _]
                  tunnel: w1317 -> [_ w1328]
                  tunnel: w1316 -> [_ w1327]
                  frame False {
                  }
                  frame True {
                    n573 = local read "AI2 Y Sum Set 2"() -> (w1332:i16)
                    n574 = call "Slower PID.vi"("process variable"=w1332, "reset?"="FB Reset Set 2", "setpoint"="FB Setpoint Set 2", "PID gains (x 2^8)"=w1328, "output range"=w1327) -> ("output"=w1330:i16)  [unwired: 10 out]
                    n575 = To Unsigned Word Integer(number=w1330) -> (unsigned 16bit integer=w1329:u16)
                  }
                }
                "BD1 amplitude 2 out" <- w1307
                n576 = Select(t=w1314, s="Trap 2 osc enable", f=i64 0) -> (s? t:f=w1313:i64)
                n577 = Add(x=w1304, y=w1313) -> (x+y=w1311:u64)
                "BD1 Frequency Out 2" <- w1311
              }
              frame 3 {
                # "Fluorescence period"
                n578 = disable-structure shown="Disabled" {
                  disable-tunnel: [w1347 _] -> w1338
                  disable-tunnel: w1337 -> [w1346 _]
                  frame Disabled {
                    # "Remember if FB was previously on/off"
                    n579 = feedback #48(FALSE) -> (w1342:bool)
                    n580 = case shown="True" w1346 {
                      tunnel: [w1349 w1365] -> w1347
                      tunnel: "BD 2 Amplitude 3" -> [w1349 _]
                      tunnel: [FALSE TRUE] -> w1343
                      tunnel: w1342 -> [_ w1351]
                      frame False {
                      }
                      frame True {
                        # "Makes it so first time FB run when turned on, the PID sees the detector intensity from the last time FB was running, rather than something near zero. Especially assuming the setpoint is not changing, this will make the FB more stable when resuming, and not overshoot the turnon intensity."
                        # "FB output range: 0 should be low, full scale is 12 bits.\nBut be careful not to go over, then higher bits just get ignored by RF board, so output will actually jump down and be unstable. Keep it under 4000 to be safe."
                        n581 = local read "Green FB Sum"() -> (w1350:i16)
                        n582 = feedback-in #49(w1350) -> ()
                        n583 = feedback #49(i16 0 ("Green FB Sum")) -> (w1353:i16)
                        n584 = Select(t=w1350, s=w1351, f=w1353) -> (s? t:f=w1352:i16)
                        n585 = Bundle("P3 2"="P3 2", "I3 2"="I3 2", "D3 2"="D3 2") -> (w1364:cluster{"P3 2":i16, "I3 2":i16, "D3 2":i16})  [unwired: 1 in]
                        n586 = Bundle("RF synth green feedback max"="RF synth green feedback max", i16 0) -> (w1356:cluster{"RF synth green feedback max":i16, i16})  [unwired: 1 in]
                        n587 = call "Slower PID.vi"("process variable"=w1352, "reset?"="Green FB Reset 2", "setpoint"="Green FB Setpoint 2", "PID gains (x 2^8)"=w1364, "output range"=w1356) -> ("output"=w1366:i16)  [unwired: 10 out]
                        n588 = To Unsigned Word Integer(number=w1366) -> (unsigned 16bit integer=w1365:u16)
                      }
                    }
                    n589 = feedback-in #48(w1343) -> ()
                  }
                  frame Enabled {
                  }
                }
              }
            }
            n590 = Split Number(x=w882) -> (hi(x)=w881:u32, lo(x)=w880:u32)
            n591 = Boolean To (0,1)(Boolean="+ phase (DIO)") -> (0, 1=w842:i16)
            n592 = Split Number(x=w881) -> (lo(x)=w879:u16)  [unwired: 1 out]
            n593 = Split Number(x=w880) -> (hi(x)=w878:u16, lo(x)=w877:u16)
            n594 = Split Number(x=w879) -> (hi(x)=w871:u8, lo(x)=w870:u8)
            n595 = Split Number(x=w878) -> (hi(x)=w869:u8, lo(x)=w868:u8)
            n596 = Split Number(x=w877) -> (hi(x)=w867:u8, lo(x)=w866:u8)
            n597 = Multiply(x=w842, y="Phase count adjustment (DIO)") -> (x*y=w838:i16)
            n598 = feedback #50(TRUE) -> (w827:bool)
            n599 = Not(x=w827) -> (.not. x?=w826:bool)
            n600 = feedback-in #50(w826) -> ()
            n601 = feedback #51(i16 0) -> (w840:i16)
            n602 = Subtract(x=w840, y=w838) -> (x-y=w839:i16)
            "DIO Relative phase" <- w839
            n603 = feedback-in #51(w839) -> ()
            n604 = Add(x=w845, y=w838) -> (x+y=w844:u32)
            n605 = Build Array "BD 1 nu Stack"(w871, w870, w869, w868, w867, w866) -> (w865:u8[])
            n606 = Not Equal?(x=w805, y=u8 3) -> (x != y?=w814:bool)
            n607 = case "Store in RF board F1 or F2" shown="True" w826 {
              tunnel: [w1037 w1041] -> w856
              tunnel: [u8 10 u8 4] -> w857
              tunnel: "Swap F1 and F2" -> [w1038 w1041]
              tunnel: "BD 2 Frequency 1" -> [_ w1040]
              tunnel: "BD 2 Frequency 2" -> [w1036 _]
              tunnel: [w1036 w1040] -> w822
              frame False {
                # "for RF synth controls\ngreen: F1/F2 stay same"
                # "F2 address (hex)"
                n608 = Not(x=w1038) -> (.not. x?=w1037:bool)
              }
              frame True {
                # "low chooses F1"
                # "F1 address (hex)"
              }
            }
            n609 = Select(t=w822, s="RF synth bd controls green", f=w821) -> (s? t:f=w820:u64)
            n610 = Split Number(x=w820) -> (hi(x)=w876:u32, lo(x)=w875:u32)
            n611 = Split Number(x=w876) -> (lo(x)=w874:u16)  [unwired: 1 out]
            n612 = Split Number(x=w875) -> (hi(x)=w873:u16, lo(x)=w872:u16)
            n613 = Split Number(x=w874) -> (hi(x)=w864:u8, lo(x)=w863:u8)
            n614 = Split Number(x=w873) -> (hi(x)=w862:u8, lo(x)=w861:u8)
            n615 = Split Number(x=w872) -> (hi(x)=w860:u8, lo(x)=w859:u8)
            n616 = feedback #52(u16 0 ("BD 2 Amplitude 3")) -> (w811:u16)
            n617 = Select(t=w811, s=w814, f=w813) -> (s? t:f=w812:u16)
            n618 = feedback-in #52(w812) -> ()
            n619 = And(x=w814, y=w817) -> (x .and. y?=w816:bool)
            n620 = Build Array "BD 2 nu Stack"(w864, w863, w862, w861, w860, w859) -> (w858:u8[])
            n621 = Select(t=w811, s=w816, f=w813) -> (s? t:f=w794:u16)
            n622 = flat-sequence "Update trap RF synth board settings to be used for the upcoming trap cycle." {
              tunnel: w858 -> [w985]
              tunnel: w865 -> [w986]
              tunnel: [w986] -> w809
              tunnel: [w985] -> w808
              tunnel: w857 -> [w987]
              tunnel: w809 -> [w989]
              tunnel: w808 -> [w988]
              tunnel: w796 -> [w1000]
              tunnel: w798 -> [w999]
              tunnel: w797 -> [w998]
              frame #0 {
                # "To possibly delay\nthese writes to very\nend of loop (for x and\ny phase adjust)"
                n623 = call "Wait8"("Count(Ticks)"="Next trap write delay (ticks)") -> ()  [unwired: 1 out]
              }
              frame #1 {
                # "Next trap RF frequency:\n\nWrite next trap cycle frequency to buffer."
                n624 = for {
                  tunnel: w989 -> [w995] mode=indexing
                  tunnel: w988 -> [w994] mode=indexing
                  tunnel: w987 -> [w992]
                  i -> [w993]
                  n625 = To Unsigned Byte Integer(number=w993) -> (unsigned 8bit integer=w990:u8)
                  n626 = Add(x=w992, y=w990) -> (x+y=w991:u8)
                  n627 = call "write to RF synth bd.vi"("Address Byte"=w991, "BD 2 Byte"=w994, "BD 1 Byte"=w995) -> ()
                }
              }
              frame #2 {
                w996 = TRUE ("Connector1/DIO15")
                # "Send udclk high\n(BD 1 and 2) to make the new frequency active in F1 or F2 word. But it won't actually be the used frequency until FSK switches to it (begining of next cycle)."
                n628 = xnode "FPGA I/O Node"("Connector1/DIO30"=w996, "Connector1/DIO29"=w996) -> ()  [unwired: 2 in, 2 out]
              }
              frame #3 {
                w997 = FALSE ("Connector1/DIO15")
                n629 = xnode "FPGA I/O Node"("Connector1/DIO30"=w997, "Connector1/DIO29"=w997) -> ()  [unwired: 2 in, 2 out]
              }
              frame #4 {
                # "Next trap RF phase offset:\n\nSet the next trap cycle amplitude to the buffer. Won't become active until udclk is set high at proper time at the begining of the next cycle."
                n630 = case shown="True" w1000 {
                  tunnel: w999 -> [_ w1001]
                  tunnel: w998 -> [_ w1002]
                  frame False {
                  }
                  frame True {
                    # "phase 1 address start"
                    n631 = for {
                      tunnel: w1001 -> [w1009] mode=indexing
                      tunnel: w1002 -> [w1008] mode=indexing
                      tunnel: u8 0 -> [w1006]
                      i -> [w1007]
                      n632 = To Unsigned Byte Integer(number=w1007) -> (unsigned 8bit integer=w1004:u8)
                      n633 = Add(x=w1006, y=w1004) -> (x+y=w1005:u8)
                      n634 = call "write to RF synth bd.vi"("Address Byte"=w1005, "BD 2 Byte"=w1008, "BD 1 Byte"=w1009) -> ()
                    }
                  }
                }
              }
              frame #5 {
                # "Prep to reset RF phase to zero at start of next cycle. Only reset BD 1. Do nothing to BD 2. This puts the settings in the buffer. A udclk high will make both this phase reset and possibly a new phase offset setting active."
                n635 = case shown="True" "RF phase reset before cycles" {
                  frame False {
                  }
                  frame True {
                    w1012 = u8 66  # BD 1 reset
                    n636 = call "write to RF synth bd.vi"("Address Byte"=u8 31, "BD 2 Byte"=u8 2, "BD 1 Byte"=w1012) -> ()
                  }
                }
              }
              frame #6 {
                # "Address"
                # "Data BD 2"
                # "Data BD 1"
                # "If phase reset wasn't chosen previously, these actions will have no affect. For both BD's, data should be binary 10, and address should be hex 1F (bin 01 1111)"
                # "This sets up the digital communication lines to restart phase accumulation (start RF running agin). It cancels out the possible phase reset. Just need to set WR DIO low then udclk DIOhigh  to make this happen. Doing this here early (and not using the usual board write function) speeds things up.\n\nRestarts RF (BD 1 only, BD2 never stopped in first place)."
                n637 = xnode "FPGA I/O Node"("Connector1/DIO0"=FALSE, "Connector1/DIO1"=FALSE, "Connector1/DIO2"=FALSE, "Connector1/DIO3"=FALSE, "Connector1/DIO4"=FALSE, "Connector1/DIO5"=FALSE, "Connector1/DIO6"=TRUE, "Connector1/DIO7"=FALSE, "Connector1/DIO8"=FALSE, "Connector1/DIO9"=TRUE, "Connector1/DIO10"=TRUE, "Connector1/DIO11"=TRUE, "Connector1/DIO12"=TRUE, "Connector1/DIO13"=TRUE, "Connector1/DIO20"=FALSE, "Connector1/DIO21"=FALSE, "Connector1/DIO22"=FALSE, "Connector1/DIO23"=FALSE, "Connector1/DIO24"=FALSE, "Connector1/DIO25"=FALSE, "Connector1/DIO26"=TRUE, "Connector1/DIO27"=FALSE) -> ()  [unwired: 22 in, 22 out]
              }
            }
            n638 = feedback #53(fxp<+,8,8> 0.0) -> (w791:fxp<+,8,8>)
            n639 = Increment(x=w791) -> (x+1=w789:fxp<+,8,8>)
            n640 = feedback-in #53(w789) -> ()
            n641 = case "Trap RF phase offset control methods" shown="3" "Phase offset method" {
              tunnel: [fxp<+,14,14> 0.0 ("Phase BD 1") w935 w950 w979] -> w799
              tunnel: "Phase Trap 1" -> [_ w936 w951 _]
              tunnel: w805 -> [_ w937 w952 w980]
              tunnel: [FALSE TRUE TRUE TRUE] -> w796
              tunnel: "Phase Trap 2" -> [_ w933 w948 _]
              tunnel: w789 -> [_ _ w947 _]
              frame 0, Default {
              }
              frame 1 {
                # "Constant increment of phase offset with each trap cycle. This results in a constant phase difference between trap cycles. \nOnly for traps 1 and 2 (set phase offset to zero for set three)."
                n642 = case shown="1, Default" w937 {
                  tunnel: w936 -> [_ _ w943]
                  tunnel: [w939 fxp<+,14,14> 0.0 w944] -> w935
                  tunnel: w933 -> [w938 _ _]
                  frame 2 {
                    n643 = feedback #54(fxp<+,14,14> 0.0) -> (w941:fxp<+,14,14>)
                    n644 = Add(x=w938, y=w941) -> (x+y=w939:fxp<+,14,14>)
                    n645 = feedback-in #54(w939) -> ()
                  }
                  frame 3 {
                  }
                  frame 1, Default {
                    n646 = feedback #55(fxp<+,14,14> 0.0) -> (w946:fxp<+,14,14>)
                    n647 = Add(x=w943, y=w946) -> (x+y=w944:fxp<+,14,14>)
                    n648 = feedback-in #55(w944) -> ()
                  }
                }
              }
              frame 2 {
                # "Changing increment of phase offset with each trap cycle. This results in a constant change in phase difference between trap cycles. \nOnly for traps 1 and 2 (set phase offset to zero for set three)."
                n649 = case shown="2" w952 {
                  tunnel: w951 -> [_ _ w962]
                  tunnel: [w953 fxp<+,14,14> 0.0 w960] -> w950
                  tunnel: w948 -> [w955 _ _]
                  tunnel: w947 -> [w956 _ w963]
                  frame 2 {
                    n650 = Multiply(x=w955, y=w956) -> (x*y=w954:fxp<+,16,16>)
                    n651 = feedback #56(fxp<+,14,14> 0.0) -> (w958:fxp<+,14,14>)
                    n652 = Add(x=w954, y=w958) -> (x+y=w953:fxp<+,14,14>)
                    n653 = feedback-in #56(w953) -> ()
                  }
                  frame 3 {
                  }
                  frame 1, Default {
                    n654 = Multiply(x=w962, y=w963) -> (x*y=w961:fxp<+,16,16>)
                    n655 = feedback #57(fxp<+,14,14> 0.0) -> (w965:fxp<+,14,14>)
                    n656 = Add(x=w961, y=w965) -> (x+y=w960:fxp<+,14,14>)
                    n657 = feedback-in #57(w960) -> ()
                  }
                }
              }
              frame 3 {
                w972 = u32 1013904223  # LCG constant C (add)
                w974 = fxp<+,21,21> 1664525.0  # LCG constant A (multiply)
                # "Set a random phase offset. Random number generated using the LCG method. Constants and method taken from NI white noise generator code (method is general though)."
                # "shift to 14 significant bits"
                n658 = feedback #58(u32 4294967295 ("seed")) -> (w969:u32)
                n659 = Multiply(x=w969, y=w974) -> (x*y=w973:u32)
                n660 = Split Number(x=w969) -> (hi(x)=w975:u16)  [unwired: 1 out]
                n661 = To Unsigned Word Integer(number=w975) -> (unsigned 16bit integer=w967:u16)
                n662 = Add(x=w973, y=w972) -> (x+y=w971:fxp<+,32,32>)
                n663 = To Unsigned Long Integer(number=w971) -> (unsigned 32bit integer=w968:u32)
                n664 = feedback-in #58(w968) -> ()
                n665 = Scale By Power Of 2(n=i8 -2 ("Uniform scale factor"), x=w967) -> (x*2^n=w976:u16)
                n666 = To Fixed-Point(number=w976) -> (fixed-point=w966:fxp<+,14,14>)  [unwired: 1 in]
                "Random phase generated" <- w966
                n667 = case shown="1, Default" w980 {
                  tunnel: [w981 fxp<+,14,14> 0.0 w983] -> w979
                  tunnel: w966 -> [w981 _ w983]
                  frame 2 {
                  }
                  frame 3 {
                  }
                  frame 1, Default {
                  }
                }
              }
            }
            n668 = To Unsigned Word Integer(number=w799) -> (unsigned 16bit integer=w804:u16)
            n669 = Split Number(x=w804) -> (hi(x)=w802:u8, lo(x)=w803:u8)
            n670 = Split Number(x=u16 0) -> (hi(x)=w800:u8, lo(x)=w801:u8)
            n671 = Build Array ("BD 1 A Stack")(w802, w803) -> (w798:u8[])
            n672 = Build Array ("BD 1 A Stack")(w800, w801) -> (w797:u8[])
          }
        }
      }
    }
  }
  n673 = while "532 nm green fluorescent laser interlacing (DO to IA 532 nm AOM ME amp)." {
    shift-right: [w1370] -> _
    shift-left: w4 -> [w1375]
    shift-right: [w1369] -> _
    shift-left: w5 -> [w1367]
    stop <- FALSE stop-if-true
    n674 = flat-sequence {
      tunnel: w1375 -> [w1378]
      tunnel: [w1377] -> w1373
      tunnel: [w1378] -> w1371
      tunnel: [w1379] -> w1368
      tunnel: w1367 -> [w1379]
      tunnel: [w1382] -> w1374
      tunnel: w1373 -> [w1382]
      tunnel: [w1381] -> w1372
      tunnel: w1371 -> [w1381]
      tunnel: w1368 -> [w1380]
      tunnel: [w1394] -> w1370
      tunnel: w1374 -> [w1413]
      tunnel: w1372 -> [w1410]
      tunnel: [w1383] -> w1369
      frame #0 {
        n675 = call "Loop Timer9"("Count(Ticks)"=w1378) -> ("Tick Count(Ticks)"=w1377:u32)
      }
      frame #1 {
        # "Then to PRL 440 amp\nOR to RF synth board FSK in"
        n676 = xnode "FPGA I/O Node"("Connector1/DIO37"=w1380, "Connector1/DIO38"=w1380, "Connector1/DIO39"=w1380, "Connector1/DIO26"=w1380, "Connector1/DIO27"=w1380, "Connector1/DIO32"=w1380) -> ()  [unwired: 6 in, 6 out]
      }
      frame #2 {
        n677 = feedback-in #59(w1413) -> ()
        n678 = feedback #59(w1413) -> (w1412:u32)
        n679 = Subtract(x=w1413, y=w1412) -> (x-y=w1411:u32)
        n680 = Subtract(x=w1411, y=w1410) -> (x-y=w1387:u32)
        n681 = Number To Boolean Array(number=w1387) -> (Boolean array=w1388:bool[])
        n682 = Or Array Elements(Boolean array=w1388) -> (logical OR=w1386:bool)
        n683 = Boolean To (0,1)(Boolean="+ phase (GI)") -> (0, 1=w1399:i16)
        n684 = Boolean To (0,1)(Boolean=w1386) -> (0, 1=w1393:i16)
        n685 = To Unsigned Byte Integer(number=w1393) -> (unsigned 8bit integer=w1390:u8)
        n686 = Multiply(x=w1399, y="Phase count adjustment (GI)") -> (x*y=w1396:i16)
        n687 = feedback #60(u8 0) -> (w1391:u8)
        n688 = Add(x=w1390, y=w1391) -> (x+y=w1389:u8)
        "GI Late Counter" <- w1389
        n689 = feedback-in #60(w1389) -> ()
        n690 = feedback #61(i16 0) -> (w1397:i16)
        n691 = Subtract(x=w1397, y=w1396) -> (x-y=w1395:i16)
        "GI Relative phase" <- w1395
        n692 = feedback-in #61(w1395) -> ()
        n693 = feedback #62(TRUE) -> (w1405:bool)
        n694 = case shown="2" "Operating Mode" {
          tunnel: [TRUE FALSE w1438] -> w1384
          tunnel: w1405 -> [_ _ w1435]
          frame 0, Default {
          }
          frame 1 {
          }
          frame 2 {
            n695 = Not(x=w1435) -> (.not. x?=w1437:bool)
            n696 = Select(t=w1437, s="Invert GI", f=w1435) -> (s? t:f=w1438:bool)
          }
        }
        n697 = Not(x=w1405) -> (.not. x?=w1402:bool)
        n698 = Select(t="Green interlace ON count", s=w1402, f="Green interlace OFF count") -> (s? t:f=w1407:u16)
        n699 = Subtract(x=w1407, y=w1387) -> (x-y=w1400:u32)
        n700 = Add(x=w1400, y=w1396) -> (x+y=w1394:u32)
        n701 = feedback-in #62(w1402) -> ()
        n702 = case shown="True" "Green long-scale interlacing" {
          tunnel: w1384 -> [w1414 w1422]
          tunnel: [w1414 w1423] -> w1383
          frame False {
          }
          frame True {
            n703 = feedback #63(i16 1) -> (w1429:i16)
            n704 = Increment(x=w1429) -> (x+1=w1428:i16)
            n705 = feedback #64("Number of ON cycles") -> (w1415:i16)
            n706 = Greater?(x=w1415, y=w1429) -> (0:w1424:bool)
            n707 = Select(t=w1428, s=w1424, f=i16 1) -> (s? t:f=w1426:i16)
            n708 = feedback-in #63(w1426) -> ()
            n709 = feedback #65(TRUE) -> (w1421:bool)
            n710 = Not(x=w1421) -> (.not. x?=w1420:bool)
            n711 = Select(t=w1421, s=w1424, f=w1420) -> (s? t:f=w1419:bool)
            n712 = Select(t="Number of ON cycles", s=w1419, f="Number of OFF cycles") -> (s? t:f=w1417:i16)
            n713 = feedback-in #64(w1417) -> ()
            n714 = feedback-in #65(w1419) -> ()
            n715 = case shown="False" w1419 {
              tunnel: [FALSE w1432] -> w1423
              tunnel: w1422 -> [_ w1432]
              frame False {
              }
              frame True {
              }
            }
          }
        }
      }
    }
  }
  n716 = while "Green excitation laser feedback measurement" {
    shift-right: [w1439] -> _
    shift-left: w4 -> [w1444]
    stop <- FALSE stop-if-true
    n717 = flat-sequence {
      tunnel: w1444 -> [w1446]
      tunnel: [w1447] -> w1442
      tunnel: [w1446] -> w1440
      tunnel: [w1454] -> w1443
      tunnel: w1442 -> [w1454]
      tunnel: [w1453] -> w1441
      tunnel: w1440 -> [w1453]
      tunnel: [w1466] -> w1439
      tunnel: w1443 -> [w1477]
      tunnel: w1441 -> [w1474]
      frame #0 {
        n718 = call "Loop Timer6"("Count(Ticks)"=w1446) -> ("Tick Count(Ticks)"=w1447:u32)
      }
      frame #1 {
        n719 = xnode "FPGA I/O Node"("Connector1/DIO35"=TRUE) -> ("Chassis2/Mod2/AI0"=w1452:i16, "Chassis2/Mod2/AI1"=w1451:i16, "Chassis2/Mod2/AI2"=w1448:i16)  [unwired: 4 in, 4 out]
        "Green FB Sum" <- w1448
        n720 = Bundle("Chassis2/Mod2/AI0"=w1452, "Chassis2/Mod2/AI1"=w1451, "Chassis2/Mod2/AI2"=w1448) -> (→"Green FB Signals":T10)  [unwired: 1 out]
      }
      frame #2 {
        n721 = feedback-in #66(w1477) -> ()
        n722 = feedback #66(w1477) -> (w1476:u32)
        n723 = Subtract(x=w1477, y=w1476) -> (x-y=w1475:u32)
        n724 = xnode "FPGA I/O Node"("Connector1/DIO35"=FALSE) -> ()  [unwired: 1 in, 1 out]
        n725 = Subtract(x=w1475, y=w1474) -> (x-y=w1456:u32)
        n726 = Subtract(x="Green FB Count", y=w1456) -> (x-y=w1470:u32)
        n727 = Number To Boolean Array(number=w1456) -> (Boolean array=w1457:bool[])
        n728 = Or Array Elements(Boolean array=w1457) -> (logical OR=w1455:bool)
        "Green FB Late?" <- w1455
        n729 = Boolean To (0,1)(Boolean="+ phase (Green FB)") -> (0, 1=w1468:i16)
        n730 = Boolean To (0,1)(Boolean=w1455) -> (0, 1=w1462:i16)
        n731 = Multiply(x=w1468, y="Phase count adjustment (Green FB)") -> (x*y=w1463:i16)
        n732 = Add(x=w1470, y=w1463) -> (x+y=w1466:u32)
        n733 = To Unsigned Word Integer(number=w1462) -> (unsigned 16bit integer=w1459:u16)
        n734 = feedback #67(i16 0) -> (w1465:i16)
        n735 = Subtract(x=w1465, y=w1463) -> (x-y=w1464:i16)
        "Green FB Relative Phase" <- w1464
        n736 = feedback-in #67(w1464) -> ()
        n737 = feedback #68(u16 0) -> (w1460:u16)
        n738 = Add(x=w1459, y=w1460) -> (x+y=w1458:u16)
        "Green Late Counter" <- w1458
        n739 = feedback-in #68(w1458) -> ()
      }
    }
  }
  n740 = while "Control APD data integration - stream to host" {
    shift-right: [w1480] -> _
    shift-left: w7 -> [w1485]
    stop <- FALSE stop-if-true
    n741 = flat-sequence {
      tunnel: w1485 -> [w1487]
      tunnel: [w1488] -> w1483
      tunnel: [w1487] -> w1481
      tunnel: [w1496] -> w1484
      tunnel: w1483 -> [w1496]
      tunnel: [w1495] -> w1482
      tunnel: w1481 -> [w1495]
      tunnel: [w1494] -> w1479
      tunnel: [w1493] -> w1478
      tunnel: [w1530] -> w1480
      tunnel: w1484 -> [w1542]
      tunnel: w1482 -> [w1539]
      tunnel: w1479 -> [w1523]
      tunnel: w1478 -> [w1522]
      frame #0 {
        n742 = call "Loop Timer4"("Count(Ticks)"=w1487) -> ("Tick Count(Ticks)"=w1488:u32)
      }
      frame #1 {
        n743 = flat-sequence {
          tunnel: [w1498] -> w1492
          tunnel: w1492 -> [w1500]
          tunnel: [w1502] -> w1491
          tunnel: [w1501] -> w1490
          tunnel: [w1500] -> w1489
          tunnel: [w1508] -> w1493
          tunnel: [w1509] -> w1494
          tunnel: w1491 -> [w1509]
          tunnel: w1490 -> [w1508]
          tunnel: w1489 -> [w1507]
          frame #0 {
            # "use two separate variable so each APD won't\nhave to wait to read"
            n744 = feedback #69(FALSE) -> (w1497:bool)
            "APD1 out state" <- w1497
            "APD2 out state" <- w1497
            n745 = Not(x=w1497) -> (.not. x?=w1498:bool)
            n746 = feedback-in #69(w1498) -> ()
          }
          frame #1 {
            n747 = local read "APD 1 Counts 1"() -> (w1506:u32)
            n748 = local read "APD 1 Counts 0"() -> (w1505:u32)
            n749 = local read "APD 2 Counts 1"() -> (w1504:u32)
            n750 = local read "APD 2 Counts 0"() -> (w1503:u32)
            n751 = Select(t=w1506, s=w1500, f=w1505) -> (s? t:f=w1502:u32)
            n752 = Select(t=w1504, s=w1500, f=w1503) -> (s? t:f=w1501:u32)
          }
          frame #2 {
            n753 = case shown="True" w1507 {
              frame False {
                w1510 = u32 0 ("APD 1 Counts 0")
                n754 = local write "APD 1 Counts 0"(w1510) -> ()
                n755 = local write "APD 2 Counts 0"(w1510) -> ()
              }
              frame True {
                w1511 = u32 0 ("APD 1 Counts 1")
                n756 = local write "APD 1 Counts 1"(w1511) -> ()
                n757 = local write "APD 2 Counts 1"(w1511) -> ()
              }
            }
          }
        }
      }
      frame #2 {
        n758 = feedback-in #70(w1542) -> ()
        n759 = feedback #70(w1542) -> (w1541:u32)
        n760 = Subtract(x=w1542, y=w1541) -> (x-y=w1540:u32)
        n761 = Subtract(x=w1540, y=w1539) -> (x-y=w1515:u32)
        n762 = case shown="True" "APD to FIFO" {
          tunnel: w1523 -> [_ w1545]
          tunnel: w1522 -> [_ w1543]
          frame False {
          }
          frame True {
            n763 = flat-sequence {
              tunnel: 0 ("Timeout") -> [w1547]
              tunnel: w1545 -> [w1548]
              tunnel: [w1547] -> w1544
              tunnel: w1544 -> [w1550]
              tunnel: w1543 -> [w1549]
              frame #0 {
                n764 = xnode ("FIFO Write")("Element"=w1548, "Timeout"=w1547) -> ()  [unwired: 1 in, 2 out]
              }
              frame #1 {
                n765 = xnode ("FIFO Write")("Element"=w1549, "Timeout"=w1550) -> ()  [unwired: 1 in, 2 out]
              }
            }
          }
        }
        n766 = Subtract(x="APD Acq Rate Count", y=w1515) -> (x-y=w1531:u32)
        n767 = Number To Boolean Array(number=w1515) -> (Boolean array=w1516:bool[])
        n768 = Or Array Elements(Boolean array=w1516) -> (logical OR=w1514:bool)
        "APD Acq Late?" <- w1514
        n769 = Boolean To (0,1)(Boolean=w1514) -> (0, 1=w1521:i16)
        n770 = To Unsigned Word Integer(number=w1521) -> (unsigned 16bit integer=w1518:u16)
        n771 = Boolean To (0,1)(Boolean="+ phase (APD Acq)") -> (0, 1=w1527:i16)
        n772 = feedback #71(u16 0) -> (w1519:u16)
        n773 = Add(x=w1518, y=w1519) -> (x+y=w1517:u16)
        "APD Acq Late Counter" <- w1517
        n774 = feedback-in #71(w1517) -> ()
        n775 = Multiply(x=w1527, y="Phase Count Adjustment (APD Acq)") -> (x*y=w1524:i16)
        n776 = Add(x=w1531, y=w1524) -> (x+y=w1530:u32)
        n777 = feedback #72(i16 0) -> (w1529:i16)
        n778 = Subtract(x=w1529, y=w1524) -> (x-y=w1526:i16)
        "APD Acq Relative Phase" <- w1526
        n779 = feedback-in #72(w1526) -> ()
        n780 = To Word Integer(number=w1523) -> (16bit integer=w1532:i16)
        n781 = To Word Integer(number=w1522) -> (16bit integer=w1533:i16)
        n782 = Multiply(x="APD 1 AO scale factor", y=w1532) -> (x*y=w1513:i16)
        n783 = Multiply(x="APD 2 AO scale factor", y=w1533) -> (x*y=w1512:i16)
        n784 = xnode "FPGA I/O Node"("Connector0/AO6"=w1513, "Connector0/AO7"=w1512) -> ()  [unwired: 2 in, 2 out]
      }
    }
  }
  n785 = disable-structure shown="Disabled" {
    disable-tunnel: w4 -> [w1551 _]
    frame Disabled {
      n786 = while "APD 3 Counter" {
        tunnel: w1551 -> [_]
        stop <- FALSE stop-if-true
        n787 = flat-sequence {
          frame #0 {
            n788 = xnode "FPGA I/O Method Node"("FPGA I/O In"=refnum<k21> "Connector0/DIO12" ("APD 2 DO"), "Timeout"=-1) -> ()  [unwired: 2 out]
          }
          frame #1 {
            n789 = local read "APD3 int gate"() -> (w1555:bool)
            n790 = case shown="True" w1555 {
              frame False {
              }
              frame True {
                n791 = local read item#-1() -> (w1556)
                n792 = case shown="True" w1556 {
                  frame False {
                    n793 = local read "APD 3 Counts 0"() -> (w1558:u32)
                    n794 = Increment(x=w1558) -> (x+1=→"APD 3 Counts 0":u32)
                  }
                  frame True {
                    n795 = local read "APD 3 Counts 1"() -> (w1560:u32)
                    n796 = Increment(x=w1560) -> (x+1=→"APD 3 Counts 1":u32)
                  }
                }
              }
            }
          }
        }
      }
    }
    frame Enabled {
    }
  }
  n797 = disable-structure shown="Disabled" {
    disable-tunnel: w4 -> [w1562 _]
    disable-tunnel: w6 -> [w1561 _]
    frame Disabled {
      n798 = while "APD 3 Gating" {
        shift-right: [w1566] -> _
        shift-left: w1562 -> [w1571]
        shift-right: [w1565] -> _
        shift-left: w1561 -> [w1563]
        stop <- FALSE stop-if-true
        n799 = flat-sequence {
          tunnel: w1571 -> [w1574]
          tunnel: [w1573] -> w1569
          tunnel: [w1574] -> w1567
          tunnel: [w1575] -> w1564
          tunnel: w1563 -> [w1575]
          tunnel: [w1578] -> w1570
          tunnel: w1569 -> [w1578]
          tunnel: [w1577] -> w1568
          tunnel: w1567 -> [w1577]
          tunnel: w1564 -> [w1576]
          tunnel: [w1599] -> w1566
          tunnel: w1570 -> [w1610]
          tunnel: w1568 -> [w1607]
          tunnel: [w1579] -> w1565
          frame #0 {
            n800 = call "Loop Timer5"("Count(Ticks)"=w1574) -> ("Tick Count(Ticks)"=w1573:u32)
          }
          frame #1 {
            # "Signal maybe then sent through \na transistor before APD"
            n801 = xnode "FPGA I/O Node"("Connector0/DIO2"=w1576) -> ()  [unwired: 1 in, 1 out]
            "APD3 int gate" <- w1576
          }
          frame #2 {
            n802 = local read "APD Gate OFF Count"() -> (w1584:u16)
            n803 = local read "APD Gate ON Count"() -> (w1585:u16)
            n804 = feedback #73(TRUE) -> (w1604:bool)
            n805 = feedback-in #74(w1610) -> ()
            n806 = feedback #74(w1610) -> (w1609:u32)
            n807 = Not(x=w1604) -> (.not. x?=w1602:bool)
            n808 = feedback-in #73(w1602) -> ()
            n809 = Subtract(x=w1610, y=w1609) -> (x-y=w1608:u32)
            n810 = Select(t=w1585, s=w1602, f=w1584) -> (s? t:f=w1606:u16)
            n811 = Subtract(x=w1608, y=w1607) -> (x-y=w1587:u32)
            n812 = Subtract(x=w1606, y=w1587) -> (x-y=w1598:u32)
            n813 = Number To Boolean Array(number=w1587) -> (Boolean array=w1588:bool[])
            n814 = Or Array Elements(Boolean array=w1588) -> (logical OR=w1586:bool)
            n815 = Boolean To (0,1)(Boolean=w1586) -> (0, 1=w1593:i16)
            n816 = Boolean To (0,1)(Boolean="+ phase (APD 3 Gate)") -> (0, 1=w1596:i16)
            n817 = To Unsigned Byte Integer(number=w1593) -> (unsigned 8bit integer=w1590:u8)
            n818 = Multiply(x=w1596, y="Phase count adjustment (APD 3 Gate)") -> (x*y=w1594:i16)
            n819 = feedback #75(u8 0) -> (w1591:u8)
            n820 = Add(x=w1590, y=w1591) -> (x+y=w1589:u8)
            "APD 3 Gate Late Counter" <- w1589
            n821 = feedback-in #75(w1589) -> ()
            n822 = Add(x=w1598, y=w1594) -> (x+y=w1599:u32)
            n823 = feedback #76(i16 0) -> (w1601:i16)
            n824 = Subtract(x=w1601, y=w1594) -> (x-y=w1600:i16)
            "APD 3 Gate Relative Phase" <- w1600
            n825 = feedback-in #76(w1600) -> ()
            n826 = local read "APD Gate Operating Mode"() -> (w1583:u8)
            n827 = case shown="2" w1583 {
              tunnel: [TRUE FALSE w1613] -> w1580
              tunnel: w1604 -> [_ _ w1613]
              frame 0, Default {
              }
              frame 1 {
              }
              frame 2 {
              }
            }
            n828 = local read "Invert APD Gate"() -> (w1582:bool)
            n829 = Not(x=w1580) -> (.not. x?=w1581:bool)
            n830 = Select(t=w1581, s=w1582, f=w1580) -> (s? t:f=w1579:bool)
          }
        }
      }
    }
    frame Enabled {
    }
  }
  n831 = disable-structure shown="Disabled" {
    disable-tunnel: w4 -> [w1616 _]
    disable-tunnel: w5 -> [w1615 _]
    frame Disabled {
      n832 = while "633 nm red  fluorescent laser interlacing (DO to IA 633 nm AOM ME amp)." {
        shift-right: [w1737] -> _
        shift-left: w1616 -> [w1742]
        shift-right: [w1736] -> _
        shift-left: w1615 -> [w1734]
        stop <- FALSE stop-if-true
        n833 = flat-sequence {
          tunnel: w1742 -> [w1745]
          tunnel: [w1744] -> w1740
          tunnel: [w1745] -> w1738
          tunnel: [w1746] -> w1735
          tunnel: w1734 -> [w1746]
          tunnel: [w1749] -> w1741
          tunnel: w1740 -> [w1749]
          tunnel: [w1748] -> w1739
          tunnel: w1738 -> [w1748]
          tunnel: w1735 -> [w1747]
          tunnel: [w1758] -> w1737
          tunnel: w1741 -> [w1778]
          tunnel: w1739 -> [w1775]
          tunnel: [w1767] -> w1736
          frame #0 {
            n834 = call "Loop Timer8"("Count(Ticks)"=w1745) -> ("Tick Count(Ticks)"=w1744:u32)
          }
          frame #1 {
            # "Then to PRL 440 amp"
            n835 = xnode "FPGA I/O Node"("Connector1/DIO32"=w1747) -> ()  [unwired: 1 in, 1 out]
          }
          frame #2 {
            n836 = feedback-in #77(w1778) -> ()
            n837 = feedback #77(w1778) -> (w1777:u32)
            n838 = Subtract(x=w1778, y=w1777) -> (x-y=w1776:u32)
            n839 = Subtract(x=w1776, y=w1775) -> (x-y=w1751:u32)
            n840 = Number To Boolean Array(number=w1751) -> (Boolean array=w1752:bool[])
            n841 = Or Array Elements(Boolean array=w1752) -> (logical OR=w1750:bool)
            n842 = Boolean To (0,1)(Boolean="+ phase (RI)") -> (0, 1=w1763:i16)
            n843 = Multiply(x=w1763, y="Phase count adjustment (RI)") -> (x*y=w1760:i16)
            n844 = Boolean To (0,1)(Boolean=w1750) -> (0, 1=w1757:i16)
            n845 = To Unsigned Byte Integer(number=w1757) -> (unsigned 8bit integer=w1754:u8)
            n846 = feedback #78(i16 0) -> (w1761:i16)
            n847 = feedback #79(u8 0) -> (w1755:u8)
            n848 = Add(x=w1754, y=w1755) -> (x+y=w1753:u8)
            "RI Late Counter" <- w1753
            n849 = feedback-in #79(w1753) -> ()
            n850 = Subtract(x=w1761, y=w1760) -> (x-y=w1759:i16)
            "RI Relative phase" <- w1759
            n851 = feedback-in #78(w1759) -> ()
            n852 = feedback #80(TRUE) -> (w1770:bool)
            n853 = case shown="2" "Red Laser Operating Mode" {
              tunnel: [TRUE FALSE w1784] -> w1767
              tunnel: w1770 -> [_ _ w1781]
              frame 0, Default {
              }
              frame 1 {
              }
              frame 2 {
                n854 = Not(x=w1781) -> (.not. x?=w1783:bool)
                n855 = Select(t=w1783, s="Invert RI", f=w1781) -> (s? t:f=w1784:bool)
              }
            }
            n856 = Not(x=w1770) -> (.not. x?=w1766:bool)
            n857 = Select(t="Red interlace ON count", s=w1766, f="Red interlace OFF count") -> (s? t:f=w1772:u16)
            n858 = Subtract(x=w1772, y=w1751) -> (x-y=w1764:u32)
            n859 = Add(x=w1764, y=w1760) -> (x+y=w1758:u32)
            n860 = feedback-in #80(w1766) -> ()
          }
        }
      }
      n861 = while "473 nm blue  fluorescent laser interlacing (DO to blue laser digital control input)." {
        shift-right: [w1633] -> _
        shift-left: w1616 -> [w1636]
        shift-right: [w1632] -> _
        shift-left: w1615 -> [w1630]
        shift-right: [w1625] -> _
        shift-left: _ -> [w1624]
        shift-right: [w1617] -> _
        shift-left: u16 0 -> [w1620]
        stop <- FALSE stop-if-true
        n862 = flat-sequence {
          tunnel: w1636 -> [w1639]
          tunnel: [w1638] -> w1635
          tunnel: [w1639] -> w1634
          tunnel: [w1642] -> w1631
          tunnel: w1630 -> [w1642]
          tunnel: w1624 -> [w1641]
          tunnel: [w1641] -> w1623
          tunnel: [w1640] -> w1621
          tunnel: w1620 -> [w1640]
          tunnel: [w1647] -> w1629
          tunnel: w1635 -> [w1647]
          tunnel: [w1646] -> w1628
          tunnel: w1634 -> [w1646]
          tunnel: w1631 -> [w1645]
          tunnel: w1623 -> [w1644]
          tunnel: [w1644] -> w1622
          tunnel: w1621 -> [w1643]
          tunnel: [w1643] -> w1619
          tunnel: [w1652] -> w1627
          tunnel: [w1651] -> w1626
          tunnel: w1628 -> [w1651]
          tunnel: w1629 -> [w1652]
          tunnel: w1622 -> [w1650]
          tunnel: w1619 -> [w1649]
          tunnel: [w1648] -> w1618
          tunnel: [w1709] -> w1633
          tunnel: w1627 -> [w1727]
          tunnel: w1626 -> [w1724]
          tunnel: [w1697] -> w1632
          tunnel: [w1695] -> w1625
          tunnel: w1618 -> [w1692]
          tunnel: [w1693] -> w1617
          frame #0 {
            n863 = call "Loop Timer7"("Count(Ticks)"=w1639) -> ("Tick Count(Ticks)"=w1638:u32)
          }
          frame #1 {
            n864 = xnode "FPGA I/O Node"("Connector1/DIO28"=w1645) -> ()  [unwired: 1 in, 1 out]
          }
          frame #2 {
            n865 = case shown="True" w1650 {
              tunnel: w1649 -> [w1653 w1655]
              tunnel: [w1653 w1654] -> w1648
              frame False {
              }
              frame True {
                n866 = flat-sequence {
                  tunnel: [w1661] -> w1658
                  tunnel: [w1660] -> w1657
                  tunnel: [w1659] -> w1656
                  tunnel: w1655 -> [w1659]
                  tunnel: w1658 -> [w1678]
                  tunnel: w1657 -> [w1675]
                  tunnel: w1656 -> [w1677]
                  tunnel: [w1676] -> w1654
                  frame #0 {
                    # "5 ns timing resolution"
                    n867 = node-c288() -> (w1664:T7)  [unwired: 1 in]
                    n868 = timed-loop {
                      timing: w1664 -> [_]
                      timing-out: [_] -> w1663
                      tunnel: "Lifetime timeout APD1" -> [w1670]
                      tunnel: [w1665] -> w1660
                      tunnel: [w1666] -> w1661
                      i -> [w1667]
                      stop <- w1669 stop-if-true
                      n869 = xnode "FPGA I/O Node"() -> ("Connector0/DIO5"=w1668:bool)  [unwired: 1 in, 1 out]
                      n870 = To Unsigned Word Integer(number=w1667) -> (unsigned 16bit integer=w1665:u16)
                      n871 = Equal?(x=w1670, y=w1665) -> (x = y?=w1666:bool)
                      n872 = Or(x=w1668, y=w1666) -> (x .or. y?=w1669:bool)
                    }
                    n873 = node-c288(w1663) -> ()
                  }
                  frame #1 {
                    n874 = Not(x=w1678) -> (.not. x?=w1679:bool)
                    n875 = case shown="True" w1679 {
                      tunnel: w1675 -> [_ w1681]
                      tunnel: w1677 -> [w1680 w1683]
                      tunnel: [w1680 w1682] -> w1676
                      frame False {
                        # "timed out, do nothing"
                      }
                      frame True {
                        # "photon detected,record time"
                        n876 = case shown="True" "Lifetime to FIFO" {
                          tunnel: w1681 -> [_ w1689]
                          tunnel: w1683 -> [w1685 w1687]
                          tunnel: [w1685 w1686] -> w1682
                          frame False {
                            # "don't record time\n(can't if doing force feedback)"
                          }
                          frame True {
                            # "number of events in fifo"
                            n877 = xnode ("FIFO Method Node")("Element"=w1689, "Timeout"=0) -> ()  [unwired: 1 in, 2 out]
                            n878 = Increment(x=w1687) -> (x+1=w1686:u16)
                          }
                        }
                        "lifetime (ticks)" <- w1681
                      }
                    }
                  }
                }
              }
            }
          }
          frame #3 {
            # "Reading fifo is tricky here since\nunknown # of events"
            # "For lifetime measurement:\nInterlacing and pulse falling"
            n879 = feedback-in #81(w1727) -> ()
            n880 = feedback #81(w1727) -> (w1726:u32)
            n881 = Subtract(x=w1727, y=w1726) -> (x-y=w1725:u32)
            n882 = Subtract(x=w1725, y=w1724) -> (x-y=w1702:u32)
            n883 = Number To Boolean Array(number=w1702) -> (Boolean array=w1703:bool[])
            n884 = Or Array Elements(Boolean array=w1703) -> (logical OR=w1701:bool)
            n885 = Boolean To (0,1)(Boolean="+ phase (BI D)") -> (0, 1=w1714:i16)
            n886 = Multiply(x=w1714, y="Phase count adjustment (BI D)") -> (x*y=w1711:i16)
            n887 = Boolean To (0,1)(Boolean=w1701) -> (0, 1=w1708:i16)
            n888 = To Unsigned Byte Integer(number=w1708) -> (unsigned 8bit integer=w1705:u8)
            n889 = feedback #82(i16 0) -> (w1712:i16)
            n890 = feedback #83(u8 0) -> (w1706:u8)
            n891 = Add(x=w1705, y=w1706) -> (x+y=w1704:u8)
            "Blue Late Counter (D)" <- w1704
            n892 = feedback-in #83(w1704) -> ()
            n893 = Subtract(x=w1712, y=w1711) -> (x-y=w1710:i16)
            "BI Relative phase (D)" <- w1710
            n894 = feedback-in #82(w1710) -> ()
            n895 = feedback #84(TRUE) -> (w1719:bool)
            n896 = case shown="2" "Blue Laser Operating Mode (D)" {
              tunnel: [TRUE FALSE w1733] -> w1697
              tunnel: w1719 -> [_ _ w1730]
              frame 0, Default {
              }
              frame 1 {
              }
              frame 2 {
                n897 = Not(x=w1730) -> (.not. x?=w1732:bool)
                n898 = Select(t=w1732, s="Invert BI (D)", f=w1730) -> (s? t:f=w1733:bool)
              }
            }
            n899 = Subtract(x=w1692, y="Lifetime events to read blue") -> (x-y=w1690:u16)
            n900 = Not(x=w1719) -> (.not. x?=w1717:bool)
            n901 = Select(t="Blue interlace ON count (D)", s=w1717, f="Blue interlace OFF count (D)") -> (s? t:f=w1721:u16)
            n902 = Subtract(x=w1721, y=w1702) -> (x-y=w1715:u32)
            n903 = Add(x=w1715, y=w1711) -> (x+y=w1709:u32)
            n904 = feedback-in #84(w1717) -> ()
            n905 = Select(t=w1690, s="Lifetime read blue fifo", f=w1692) -> (s? t:f=w1693:u16)
            "lifetime events in fifo" <- w1693
            n906 = Equal?(x="Blue Laser Operating Mode (D)", y=u8 2) -> (x = y?=w1698:bool)
            n907 = Not(x=w1697) -> (.not. x?=w1696:bool)
            n908 = And(x=w1696, y=w1698) -> (x .and. y?=w1695:bool)
          }
        }
      }
    }
    frame Enabled {
    }
  }
